vi "pointReactorSimulator.vi"() -> ()   [LabVIEW 2020]
doc: "本程序通过点堆动力学模型模拟核电站的反应堆运行状态。"
uses:
  <vilib>/Instr/_visa.llb/VISA Find Search Mode.ctl
  <vilib>/Utility/sysdir.llb/System Directory Type.ctl
  <vilib>/Utility/error.llb/DialogType.ctl
  Utility/Typedefs/KE622x -- Instrument Type.ctl
  Configure/Source/Typedefs/KE622x -- Voltage Limit.ctl
  Configure/Source/Typedefs/KE622x -- Current Range.ctl
  Configure/Source/Typedefs/KE622x -- Current Ranges.ctl
  <vilib>/DAQmx/write.llb/DAQmx Write (Counter 1D Frequency 1Chan NSamp).vi
  <vilib>/DAQmx/write.llb/DAQmx Write (Analog DBL 1Chan 1Samp).vi
  <vilib>/Analysis/polynomials.llb/Scalar Polynomial Evaluation (DBL).vi
  <vilib>/Instr/_visa.llb/VISA Configure Serial Port (Instr).vi
  <vilib>/DAQmx/create/channels.llb/DAQmx Create Channel (CO-Pulse Generation-Frequency).vi
  <vilib>/DAQmx/configure/timing.llb/DAQmx Timing (Implicit).vi
  <vilib>/DAQmx/create/channels.llb/DAQmx Create Channel (AO-Voltage-Basic).vi
  <vilib>/DAQmx/miscellaneous.llb/DAQmx Fill In Error Info.vi
  TcpModbus_SlaveServer/MB Slave Init (poly).vi
  TcpModbus_SlaveServer/MB Globals.vi
  TcpModbus_SlaveServer/MB Slave Read Holding Registers (poly).vi
  TcpModbus_SlaveServer/MB Slave Write Input Registers (poly).vi
  PointReactorDll.dll
  <vilib>/Analysis/NI_AALPro.lvlib
  Keithley 622x.lvlib
  <resource>/objmgr/daqmx.rc
panel:
  out "KE6220_2":bool
  in  "物理参数设置":bool
  in  "endian Switch":bool
  out "反应性仪输出电压":dbl[](array[numeric])
  out "输出电压":dbl[](array[numeric])
  in  "输出电流 (A)":dbl
  in  "电压输出选择":bool
  out "中子注量率 (n/cm2·s)":dbl
  out "硼总价值 (pcm)":dbl
  out "棒总价值 (pcm)":dbl
  out "硼浓度 indicator":dbl
  in  "硼浓度 (ppm)":dbl(slide)=1.0 scale=0.0..2000.0
  out "运行时间 (s)":dbl
  in  "TCP端口号":u16=502 min=1 max=9999
  out "堆芯反应性(硼+棒) (pcm)":dbl
  out "keff":dbl
  in  "S棒组":dbl(slide)=100.0 min=0.0 max=225.0 scale=0.0..225.0
  in  "A棒组":dbl(slide)=100.0 min=0.0 max=225.0 scale=0.0..225.0
  in  "B棒组":dbl(slide)=100.0 min=0.0 max=225.0 scale=0.0..225.0
  in  "C棒组":dbl(slide)=100.0 min=0.0 max=225.0 scale=0.0..225.0
  in  "堆芯后备反应性 (pcm)":dbl
  out "S棒价值":dbl
  out "A棒价值":dbl
  out "B棒价值":dbl
  out "C棒价值":dbl
  out "D棒价值":dbl
  out "中子注量曲线":dbl(graph) caption="Waveform Chart - Dark"
  in  "D棒组":dbl(slide)=100.0 min=0.0 max=225.0 scale=0.0..225.0
  out "CARD":bool
  out "KE6220_1":bool
  out "COM2":bool
  out "COM1":bool
  in  "VO 4":u16(ring)=3 items=["D棒位 (step)", "C棒位 (step)", "B棒位 (step)", "A棒位 (step)", "S棒位 (step)", "硼浓度 (ppm)", "中间量程电流 (A)", "源量程计数 (CPS)"]
  in  "VO 3":u16(ring)=2 items=["D棒位 (step)", "C棒位 (step)", "B棒位 (step)", "A棒位 (step)", "S棒位 (step)", "硼浓度 (ppm)", "中间量程电流 (A)", "源量程计数 (CPS)"]
  in  "VO 2":u16(ring)=1 items=["D棒位 (step)", "C棒位 (step)", "B棒位 (step)", "A棒位 (step)", "S棒位 (step)", "硼浓度 (ppm)", "中间量程电流 (A)", "源量程计数 (CPS)"]
  in  "VO 1":u16(ring) items=["D棒位 (step)", "C棒位 (step)", "B棒位 (step)", "A棒位 (step)", "S棒位 (step)", "硼浓度 (ppm)", "中间量程电流 (A)", "源量程计数 (CPS)"]
  in  "电信号输出设置":bool
  in  "TCP服务器开":bool
  out "Holding Registers":sgl[](array[numeric]) caption="Holding Registers (Read&Write)"
  out "Coils":bool[](array[boolean]) caption="Coils (Master can write coils)"
  in  "电流输出选择":u16(ring) items=["中间量程电流", "功率量程电流"]
  out "棒位与硼浓度":dbl[](array[numeric])
  in  "反应性控制方式":bool
  in  "归零":bool
  in  "棒速(step/min)":dbl=72.0 min=1.0 max=10000.0 step=1.0 format="%#.3g"
  in  "开始降棒":bool
  in  "降棒选择":u16(ring) items=["D棒组", "C棒组", "B棒组", "A棒组", "S棒组"]
  in  "细分时间 (ms)":u32=100 min=10 max=1000 step=1
  in  "开始":bool
  in  "时间比例尺":dbl(knob)=1.0 min=0.1 max=1000.0 step=0.1 scale=0.1..1000.0
  out "功率量程 (A)":dbl(slide) scale=2.875e-12..0.00023 scale format="%#_6e"
  out "中间量程 (A)":dbl(slide) scale=1e-11..0.0008 scale format="%#_6e"
  out "源量程 (CPS)":dbl(slide) scale=1.0..1000000.0 scale format="%#_6f"
  out "%FP":dbl(slide) scale=2e-09..200.0 scale format="%#_6e"
  out "中子注量率":dbl(slide) scale=0.1..10000000000.0 scale format="%#_6e"
  in  "时间步长 (s)":dbl=0.1
  in  "初始注量率 (n/cm2·s)":dbl=1.0
  in  "堆芯反应性 (pcm)":dbl
  in  "停止":bool
  in  "初始反应性 (pcm)":dbl
  # "反应性仪测试用点堆模拟器"
  # "探测器"
  # "手输"
  # "棒硼"
  # "1.25E+5 n/cm2·s\n——"
  # "——\n1.25E+2 n/cm2·s"
  # "——  1.25E-1 n/cm2·s"
  # "硬件测试"
  # "小端"
  # "0-10V"
  # "1-5V"
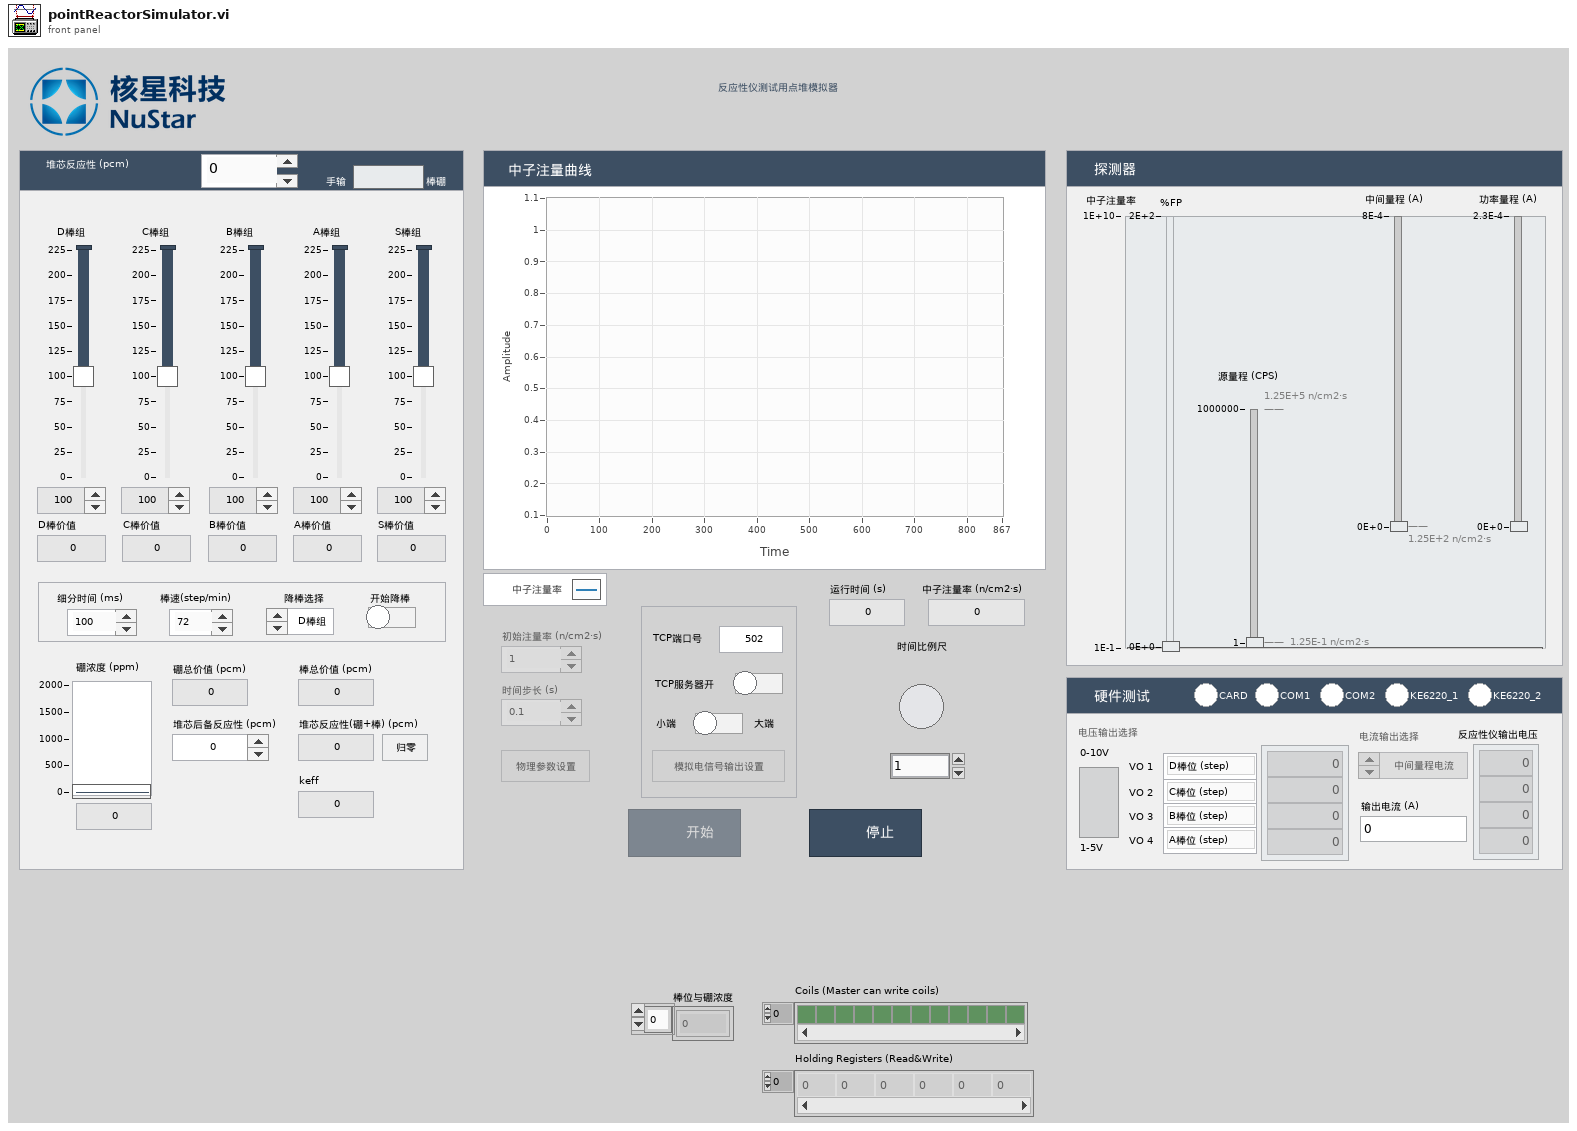
[diagram p1: front panel]
types:
  T1 = enum8{"Enabled", "Disabled", "Disabled and Grayed Out"}
  T2 = typedef "System Directory Type.ctl" = i32
  T3 = typedef "VISA Find Search Mode.ctl" = u32
  T4 = enum16{"open", "open or create", "create or replace", "create", "open (read only)"}
  T5 = typedef "DialogType.ctl" = u16
  T6 = typedef "Keithley 622x.lvlib/KE622x -- Voltage Limit.ctl" = dbl
  T7 = typedef "Keithley 622x.lvlib/KE622x -- Instrument Type.ctl" = enum16{"KE6220", "KE6221"}
  T8 = typedef "Keithley 622x.lvlib/KE622x -- Current Range.ctl" = cluster{"Auto Range?":bool, "Man / Selected\nRange":T9}
  T9 = typedef "Keithley 622x.lvlib/KE622x -- Current Ranges.ctl" = enum16{"2nA", "20nA", "200nA", "2uA", "20uA", "200uA", "2mA", "20mA", "100mA"}
  T10 = enum32{"invalid app kind", "Development System", "Run Time System", "Student Edition", "Embedded LabVIEW", "Evaluation", "Custom"}
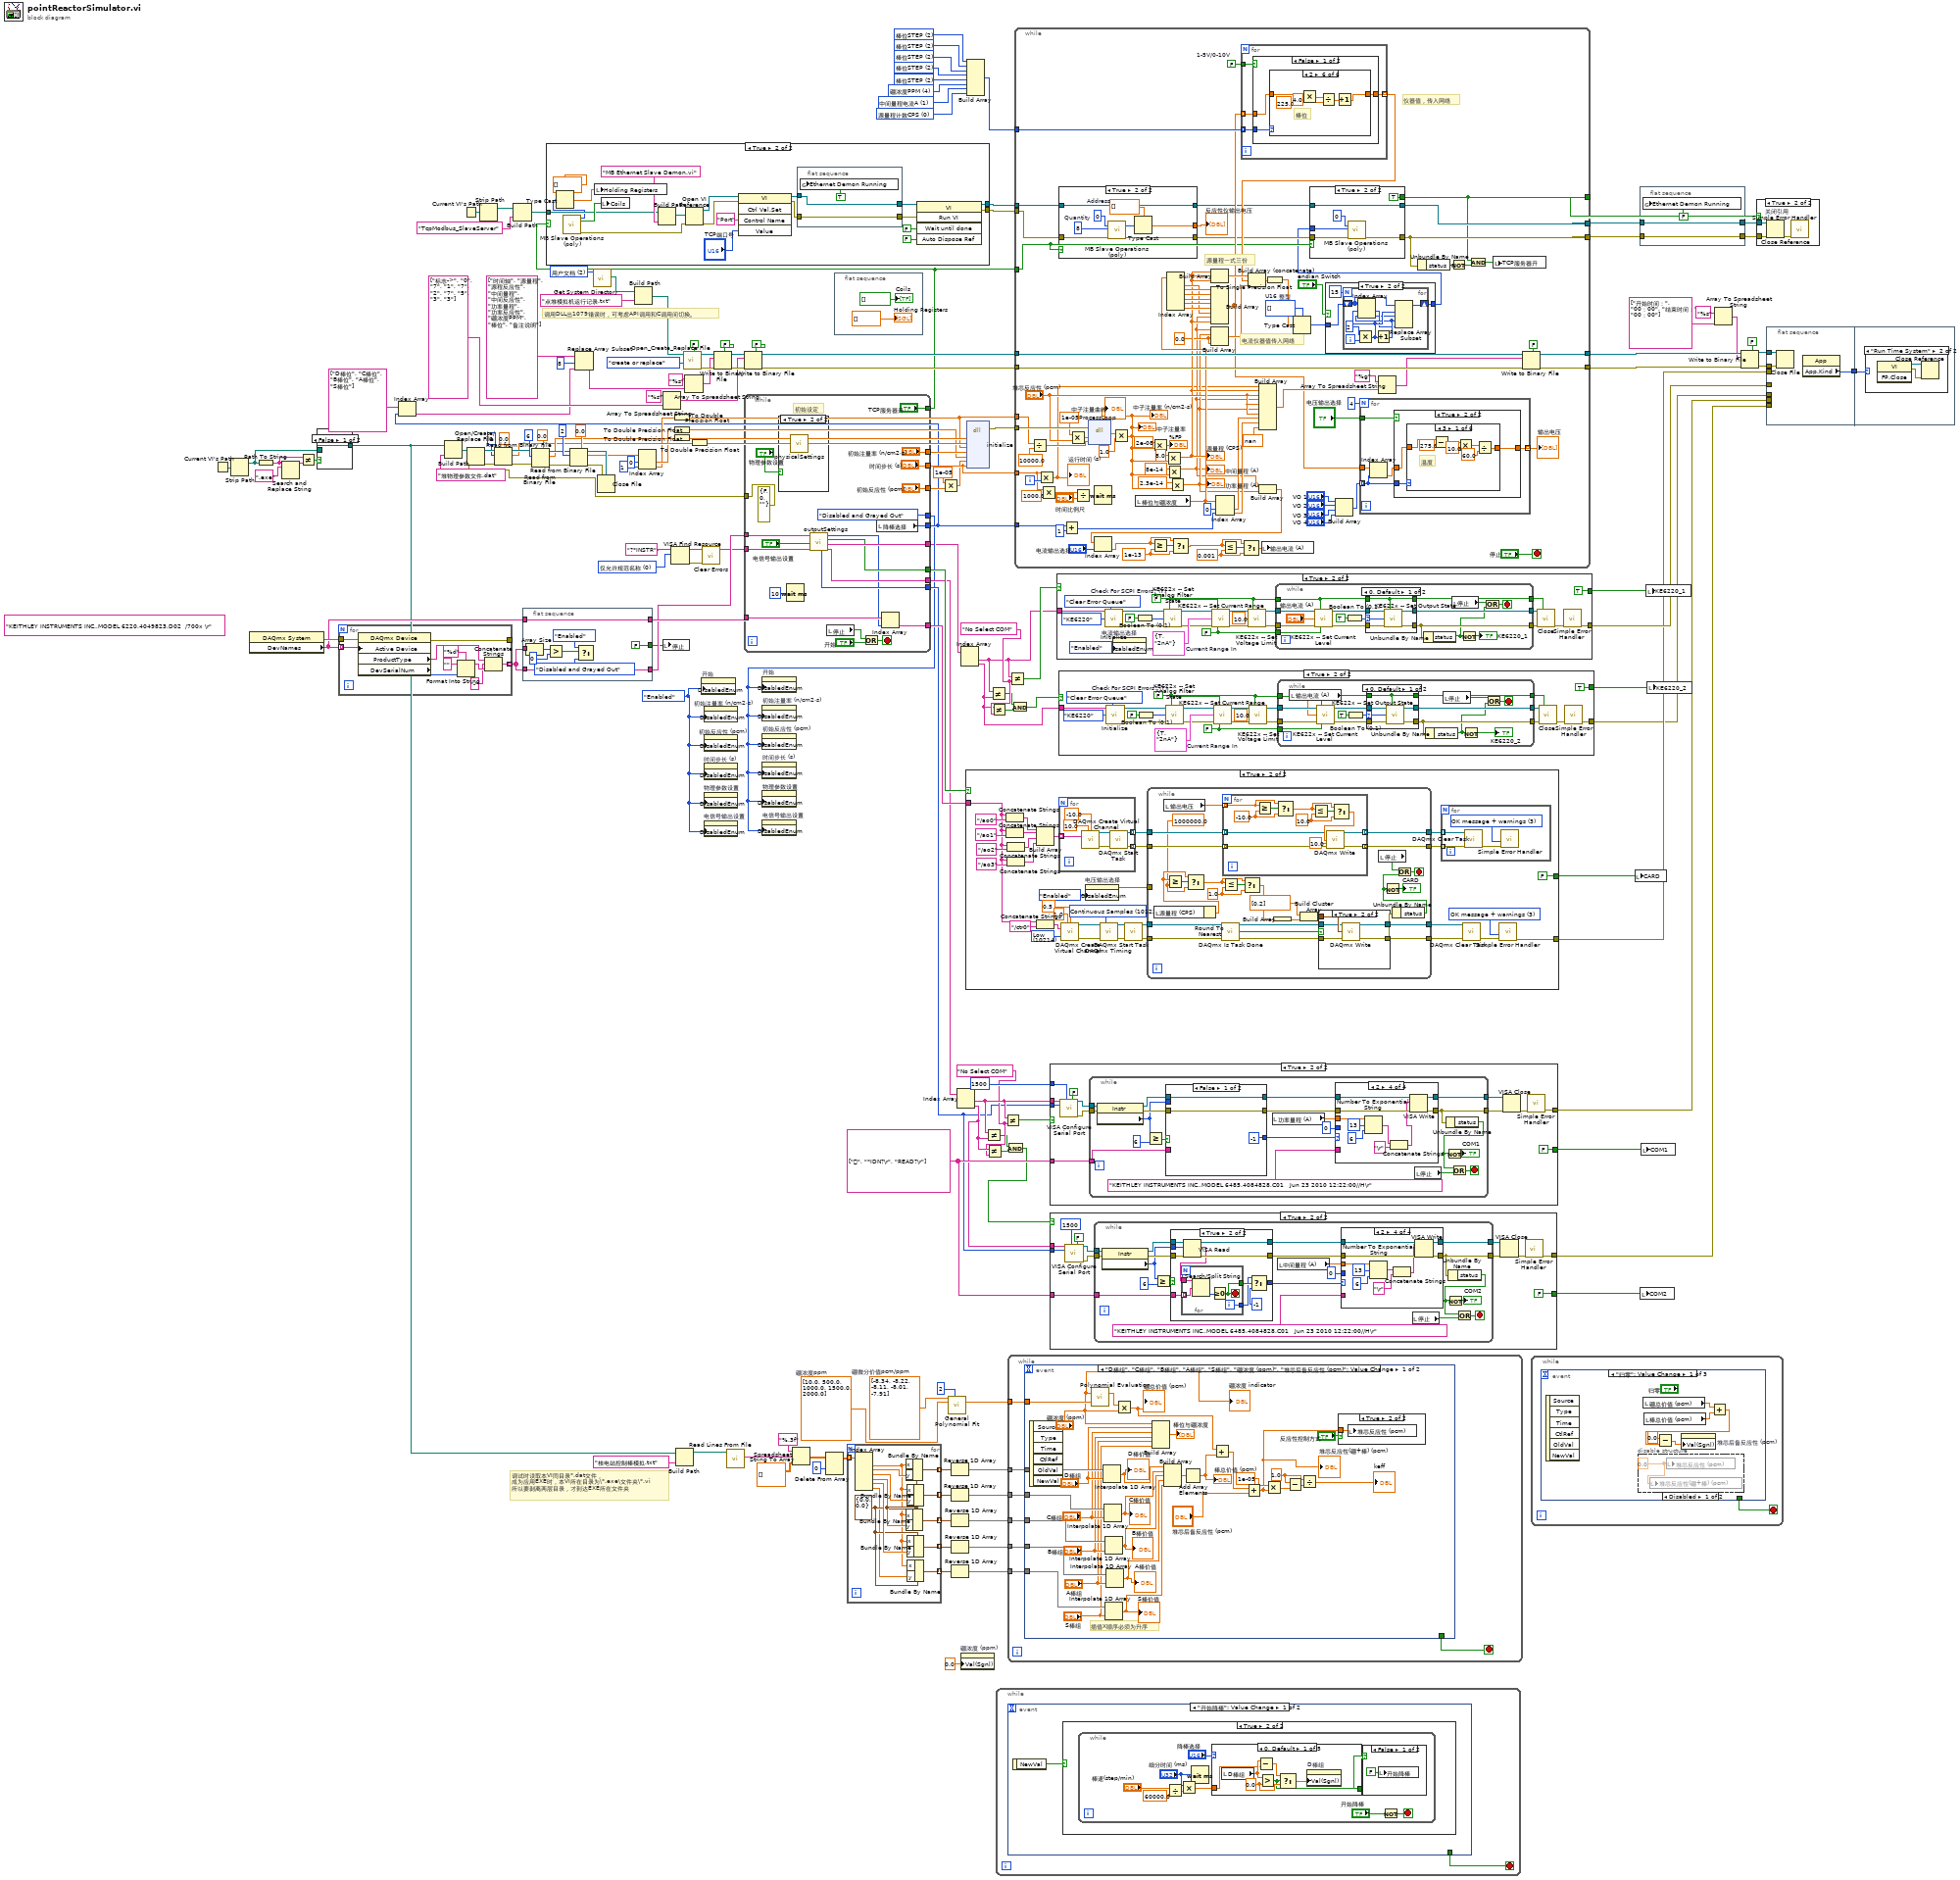
[diagram p0: block diagram]
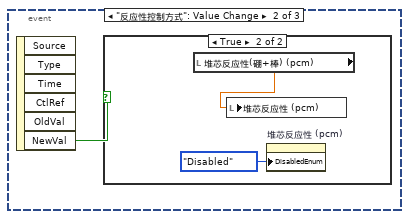
[diagram p3: hidden frame]
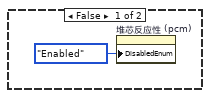
[diagram p4: hidden frame]
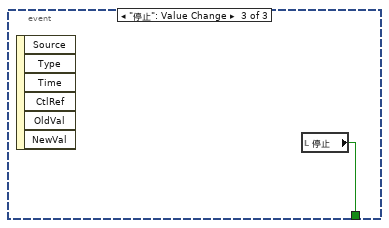
[diagram p5: hidden frame]
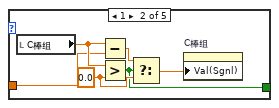
[diagram p8: hidden frame]
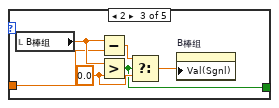
[diagram p9: hidden frame]
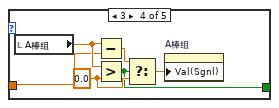
[diagram p10: hidden frame]
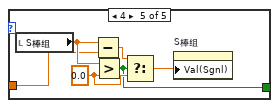
[diagram p11: hidden frame]
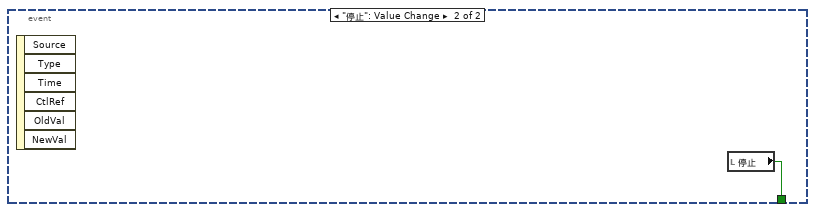
[diagram p12: hidden frame]
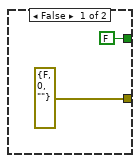
[diagram p13: hidden frame]
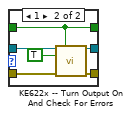
[diagram p14: hidden frame]
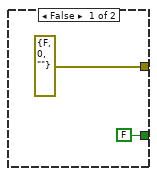
[diagram p15: hidden frame]
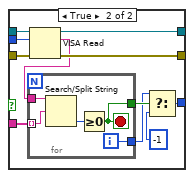
[diagram p16: hidden frame]
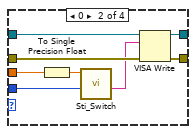
[diagram p18: hidden frame]
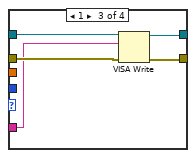
[diagram p19: hidden frame]
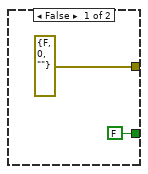
[diagram p20: hidden frame]
diagram:
  w3 = T1."Enabled" ("禁用")
  w11 = "No Select COM" ("新元素/子数组")
  (unwired) "KEITHLEY INSTRUMENTS INC.,MODEL 6220,4049823,D02  /700x \r" ("y")
  w17 = T2 2 items=["用户目录"=0, "用户桌面"=1, "用户文档"=2, "用户应用程序数据"=3, "用户设置"=4, "用户临时目录"=5, "公共文档"=6, "公共应用程序数据"=7, "公共设置"=8, "公共缓存"=13, "系统核心库"=9, "系统安装库"=10, "应用程序文件"=11, "启动盘根目录"=12] ("system directory type")
  w37 = "No Select COM" ("新元素/子数组")
  w42 = string[] ["", "*IDN?\r", "READ?\r"] ("添加的数组")
  w52 = u16 0 items=["源量程计数CPS", "中间量程电流A", "棒位STEP", "温度(摄氏度)", "硼浓度PPM", "P2电压信号"] ("P2-8")
  w51 = u16 1 items=["源量程计数CPS", "中间量程电流A", "棒位STEP", "温度(摄氏度)", "硼浓度PPM", "P2电压信号"] ("P2-7")
  w50 = u16 4 items=["源量程计数CPS", "中间量程电流A", "棒位STEP", "温度(摄氏度)", "硼浓度PPM", "P2电压信号"] ("P2-6")
  w49 = u16 2 items=["源量程计数CPS", "中间量程电流A", "棒位STEP", "温度(摄氏度)", "硼浓度PPM", "P2电压信号"] ("P2-5")
  w48 = u16 2 items=["源量程计数CPS", "中间量程电流A", "棒位STEP", "温度(摄氏度)", "硼浓度PPM", "P2电压信号"] ("P2-4")
  w47 = u16 2 items=["源量程计数CPS", "中间量程电流A", "棒位STEP", "温度(摄氏度)", "硼浓度PPM", "P2电压信号"] ("P2-3")
  w46 = u16 2 items=["源量程计数CPS", "中间量程电流A", "棒位STEP", "温度(摄氏度)", "硼浓度PPM", "P2电压信号"] ("P2-2")
  w45 = u16 2 items=["源量程计数CPS", "中间量程电流A", "棒位STEP", "温度(摄氏度)", "硼浓度PPM", "P2电压信号"] ("P2-1")
  w65 = T3 0 items=["仅允许规范名称"=0, "只允许别名"=2, "包含匹配别名"=3, "包含所有别名"=4] ("Search Mode")
  w91 = dbl[] [-8.34, -8.22, -8.11, -8.01, -7.91]  # 硼微分价值pcm/ppm
  w90 = dbl[] [10.0, 500.0, 1000.0, 1500.0, 2000.0]  # 硼浓度ppm
  # "调试时读取本VI同目录*.dat文件，\n成为应用EXE时，本VI所在目录为\\*.exe\\文件夹\\*.vi\n所以要剥离两层目录，才到达EXE所在文件夹"
  # "调用DLL出1079错误时，可考虑API调用和C调用间切换。"
  n1 = Current VI's Path() -> (path=w125:path)
  n2 = Strip Path(path=w125) -> (stripped path=w120:path)  [unwired: 1 out]
  n3 = property class="DAQmx System"() -> (error out=w71:errorcluster, "DevNames"=w69:tag[])  [unwired: 2 in, 1 out]
  n4 = Path To String(path=w120) -> (string=w122:string)
  n5 = Search and Replace String(input string=w122, search string=".exe" ("搜索字符串")) -> (result string=w123:string)  [unwired: 6 in, 3 out]
  n6 = Not Equal?(x=w122, y=w123) -> (x != y?=w121:bool)
  n7 = case shown="False" w121 {
    tunnel: w120 -> [w163 w165]
    tunnel: [w163 w164] -> w19
    frame False {
    }
    frame True {
      n8 = Strip Path(path=w165) -> (stripped path=w164:path)  [unwired: 1 out]
    }
  }
  n9 = for {
    tunnel: w69 -> [w175] mode=indexing
    tunnel: w71 -> [w174]
    tunnel: [w173] -> _
    tunnel: [w166] -> w70 mode=indexing
    n10 = property class="DAQmx Device"(error in=w174, "Active Device"=w175) -> (error out=w173:errorcluster, "ProductType"=w169:string, "DevSerialNum"=w170:u32)  [unwired: 1 in, 1 out]
    n11 = Format Into String(format string="%d" ("格式字符串"), initial string="" ("初始字符串"), w170) -> (resulting string=w168:string)  [unwired: 1 in, 1 out]
    n12 = Concatenate Strings(w169, "-" ("字符串"), w168) -> (w166:string)
  }
  n13 = Build Path(base path=w19, name or relative path="堆物理参数文件.dat") -> (appended path=w126:path)
  n14 = Current VI's Path() -> (path=w57:path)
  n15 = Strip Path(path=w57) -> (stripped path=w56:path)  [unwired: 1 out]
  n16 = Build Path ("创建路径")(base path=w56, name or relative path="TcpModbus_SlaveServer" ("搜索字符串")) -> (appended path=w55:path)
  n17 = flat-sequence {
    tunnel: w70 -> [w184]
    tunnel: [w179] -> w43
    tunnel: w70 -> [w179]
    tunnel: w69 -> [w178]
    tunnel: [w178] -> w68
    tunnel: [FALSE ("停止")] -> w28
    frame #0 {
      n18 = Array Size(array=w184) -> (size(s)=w183:i32)
      n19 = Greater?(x=w183, y=0) -> (0:w180:bool)
      n20 = Select(t=T1."Enabled" ("禁用"), s=w180, f=T1."Disabled and Grayed Out" ("禁用")) -> ()  [unwired: 1 out]
    }
  }
  n21 = call <vilib>:"Get System Directory.vi"("system directory type"=w17) -> ("system directory"=w18:path)  [unwired: 10 in]
  n22 = Build Path(base path=w18, name or relative path="点堆模拟机运行记录.txt") -> (appended path=w135:path)
  n23 = local write "停止"(w28) -> ()
  n24 = Array To Spreadsheet String(array=string[] ["标志->", "0", "7", "1", "7", "2", "7", "5", "3", "3"] ("添加的数组"), 3:"%s" ("format string")) -> (spreadsheet string=w148:string)  [unwired: 1 in]
  n25 = VISA Find Resource(10:w65, 11:"?*INSTR" ("表达式(\"?*\")")) -> (0:w58:errorcluster, 3:w14:string[])  [unwired: 1 in, 1 out]
  n26 = Build Path(base path=w19, name or relative path="核电站控制棒模拟.txt") -> (appended path=w108:path)
  n27 = call <vilib>:"Open_Create_Replace File.vi"("advisory dialog? (display:T)"=FALSE, "function (open:0)"=T4."create or replace", "file path"=w135) -> ("error out"=w155:errorcluster, "refnum"=w156:refnum<file>)  [unwired: 5 in, 2 out]
  n28 = property on="开始" class="Bool"("DisabledEnum"=w3) -> ()  [unwired: 2 in, 2 out]
  n29 = call <vilib>:"Clear Errors.vi"("error in (no error)"=w58) -> ()  [unwired: 5 in, 2 out]
  n30 = property on="初始注量率 (n/cm2·s)" class="DigNum (strict)"("DisabledEnum"=w3) -> ()  [unwired: 2 in, 2 out]
  n31 = property on="初始反应性 (pcm)" class="DigNum (strict)"("DisabledEnum"=w3) -> ()  [unwired: 2 in, 2 out]
  n32 = property on="时间步长 (s)" class="DigNum (strict)"("DisabledEnum"=w3) -> ()  [unwired: 2 in, 2 out]
  n33 = property on="物理参数设置" class="Bool"("DisabledEnum"=w3) -> ()  [unwired: 2 in, 2 out]
  n34 = property on="电信号输出设置" class="Bool"("DisabledEnum"=w3) -> ()  [unwired: 2 in, 2 out]
  n35 = call <vilib>:"Read Lines From File.vi"("file path (dialog if empty)"=w108) -> ("line string"=w105:string)  [unwired: 5 in, 3 out]
  n36 = while {
    tunnel: ["初始注量率 (n/cm2·s)"] -> w161
    tunnel: ["时间步长 (s)"] -> w160
    tunnel: ["初始反应性 (pcm)"] -> w132
    tunnel: [w200] -> w63
    tunnel: [w196] -> w8
    tunnel: [w195] -> w72
    tunnel: w68 -> [w203]
    tunnel: [w202] -> w67
    tunnel: ["TCP服务器开"] -> w60
    tunnel: w14 -> [w198]
    tunnel: [w193] -> w53
    tunnel: [w197] -> w33
    tunnel: w43 -> [w199]
    tunnel: [T1."Disabled and Grayed Out" ("禁用")] -> w15
    tunnel: [errorcluster {"status"=FALSE, "code"=0, "source"=""} ("error in")] -> w16
    stop <- w189 stop-if-true
    # "初始设定"
    n37 = case shown="True" "物理参数设置" {
      frame False {
      }
      frame True {
        n38 = call "physicalSettings.vi"() -> ()  [unwired: 1 in]
      }
    }
    n39 = Wait (ms)(milliseconds to wait=u32 10) -> ()  [unwired: 1 out]
    n40 = call "outputSettings.vi"("所有串口"=w198, "执行:调用时显示前面板"="电信号输出设置", "电压脉冲卡选择"=w199) -> ("串口电流服务选定口"=w193:string[], "电流源串口选定"=w196:string[], "电压脉冲开关 2"=w195:bool, "电压脉冲卡选"=w192:u16, "波特率set"=w197:u32)  [unwired: 4 in]
    n41 = local read "停止"() -> (w191:bool)
    n42 = Or(x=w191, y="开始") -> (x .or. y?=w189:bool)
    n43 = local read "降棒选择"() -> (w200:u16)
    n44 = Index Array(array=w203, index=w192) -> (element=w202:tag)
  }
  n45 = Index Array(array=string[] ["D棒位", "C棒位", "B棒位", "A棒位", "S棒位"] ("添加的数组"), index=w63) -> (element=w74:string)
  n46 = Open/Create/Replace File(file path (use dialog)=w126, error in=w16) -> (refnum out=w131:refnum<file>, error out=w130:errorcluster)  [unwired: 4 in, 1 out]
  n47 = Read from Binary File(5:sgl 0.0 ("byte stream type"), 8:w130, 10:6 ("count"), 11:w131) -> (0:w116:errorcluster, 2:w82:sgl[], 3:w117:refnum<file>)  [unwired: 2 in, 1 out]
  n48 = Read from Binary File(5:sgl 0.0 ("byte stream type"), 8:w116, 10:6 ("count"), 11:w117) -> (0:w112:errorcluster, 2:w84:sgl[], 3:w113:refnum<file>)  [unwired: 2 in, 1 out]
  n49 = case shown="True" w60 {
    tunnel: [refnum<vi> refnum w216] -> w62
    tunnel: [errorcluster {"status"=FALSE, "code"=0, "source"=""} ("error out") w215] -> w61
    tunnel: w55 -> [_ w214]
    frame False {
    }
    frame True {
      n50 = call-poly "MB Slave Operations (poly).vi"() -> ("Holding Registers"=w213:u16[], "Coils"=w224:bool[], "error out"=w222:errorcluster)  [unwired: 1 in, 16 out]
      n51 = Type Cast(type=sgl[] [] ("添加的数组"), x=w213) -> (*(type *) &x=w212:sgl[])
      n52 = local write "Holding Registers"(w212) -> ()
      n53 = local write "Coils"(w224) -> ()
      n54 = Build Path ("创建路径")(base path=w214, name or relative path="MB Ethernet Slave Demon.vi") -> (appended path=w210:path)
      n55 = Open VI Reference(vi path=w210, error in (no error)=w222) -> (vi reference=w219:refnum<vi>, error out=w220:errorcluster)  [unwired: 4 out]
      n56 = invoke class="VI" method="Ctrl Val.Set"(reference=w219, error in=w220, "Control Name"="Port", "Value"="TCP端口号") -> (reference out=w227:refnum<vi>, error out=w226:errorcluster)  [unwired: 1 in, 3 out]
      n57 = flat-sequence {
        tunnel: [w231] -> w223
        tunnel: w226 -> [w231]
        tunnel: [w229] -> w225
        tunnel: w227 -> [w229]
        frame #0 {
          n58 = global write "MB Globals.vi" "Ethernet Demon Running"(TRUE ("Slave Demon Running")) -> ()
        }
      }
      n59 = invoke class="VI" method="Run VI"(reference=w225, error in=w223, "Wait until done"=FALSE, "Auto Dispose Ref"=FALSE) -> (reference out=w216:refnum<vi>, error out=w215:errorcluster)  [unwired: 1 in, 3 out]
    }
  }
  n60 = Read from Binary File(5:sgl 0.0 ("byte stream type"), 8:w112, 10:2 ("count"), 11:w113) -> (0:w110:errorcluster, 2:w87:sgl[], 3:w111:refnum<file>)  [unwired: 2 in, 1 out]
  n61 = Replace Array Subset(array=string[] ["时间轴", "源量程", "源程反应性", "中间量程", "中间反应性", "功率量程", "功率反应性", "硼浓度PPM", "棒位", "备注说明"] ("添加的数组"), new element=w74, index=8 ("索引")) -> (w73:string[])
  n62 = Close File(refnum=w111, error in=w110) -> ()  [unwired: 2 out]
  n63 = Index Array(array=w87, index #1=0 ("索引"), index #2=1 ("索引")) -> (element #1=w80:sgl, element #2=w78:sgl)
  n64 = To Double Precision Float(number=w78) -> (double precision float=w77:dbl)
  n65 = To Double Precision Float(number=w80) -> (double precision float=w79:dbl)
  n66 = To Double Precision Float(number=w84) -> (double precision float=w83:dbl[])
  n67 = Array To Spreadsheet String(array=w73, 3:"%s" ("format string")) -> (spreadsheet string=w153:string)  [unwired: 1 in]
  n68 = To Double Precision Float(number=w82) -> (double precision float=w81:dbl[])
  n69 = Write to Binary File(file (use dialog)=w156, data=w153, error in=w155, 5:FALSE ("预置数组或字符串大小？(T)")) -> (refnum out=w151:refnum<file>, error out=w150:errorcluster)  [unwired: 2 in, 1 out]
  n70 = Write to Binary File(file (use dialog)=w151, data=w148, error in=w150, 5:FALSE ("预置数组或字符串大小？(T)")) -> (refnum out=w146:refnum<file>, error out=w145:errorcluster)  [unwired: 2 in, 1 out]
  n71 = property on="开始" class="Bool"("DisabledEnum"=w15) -> ()  [unwired: 2 in, 2 out]
  n72 = property on="初始注量率 (n/cm2·s)" class="DigNum (strict)"("DisabledEnum"=w15) -> ()  [unwired: 2 in, 2 out]
  n73 = property on="初始反应性 (pcm)" class="DigNum (strict)"("DisabledEnum"=w15) -> ()  [unwired: 2 in, 2 out]
  n74 = property on="时间步长 (s)" class="DigNum (strict)"("DisabledEnum"=w15) -> ()  [unwired: 2 in, 2 out]
  n75 = property on="物理参数设置" class="Bool"("DisabledEnum"=w15) -> ()  [unwired: 2 in, 2 out]
  n76 = property on="电信号输出设置" class="Bool"("DisabledEnum"=w15) -> ()  [unwired: 2 in, 2 out]
  n77 = Spreadsheet String To Array ("电子表格字符串至数组转换")(format string="%.3f" ("format (%.3f)"), spreadsheet string=w105, array type (2D Dbl)=dbl[][] [] ("type (empty)")) -> (array=w104:dbl[][])  [unwired: 1 in]
  n78 = Delete From Array(array=w104, index (row)=0 ("索引 (行)")) -> (array with subset deleted=w102:dbl[][])  [unwired: 2 in, 1 out]
  n79 = flat-sequence {
    frame #0 {
      "Coils" <- bool[] [] ("Coils")
      "Holding Registers" <- sgl[] [] ("Holding Registers")
    }
  }
  n80 = for {
    tunnel: w102 -> [w246] mode=indexing
    tunnel: [w244] -> w101 mode=indexing
    tunnel: [w240] -> w99 mode=indexing
    tunnel: [w239] -> w98 mode=indexing
    tunnel: [w238] -> w97 mode=indexing
    tunnel: [w236] -> w93 mode=indexing
    w237 = cluster{"x":dbl, "y":dbl} {"x"=0.0, "y"=0.0} ("输入簇")
    n81 = Index Array(array=w246) -> (element #1=w234:dbl, element #2=w245:dbl, element #3=w243:dbl, element #4=w242:dbl, element #5=w241:dbl, element #6=w235:dbl)  [unwired: 6 in]
    n82 = Bundle By Name(cluster=w237, "x"=w234, "y"=w245) -> (w244:cluster{"x":dbl, "y":dbl})
    n83 = Bundle By Name(cluster=w237, "x"=w234, "y"=w242) -> (w239:cluster{"x":dbl, "y":dbl})
    n84 = Bundle By Name(cluster=w237, "x"=w234, "y"=w243) -> (w240:cluster{"x":dbl, "y":dbl})
    n85 = Bundle By Name(cluster=w237, "x"=w234, "y"=w241) -> (w238:cluster{"x":dbl, "y":dbl})
    n86 = Bundle By Name(cluster=w237, "x"=w234, "y"=w235) -> (w236:cluster{"x":dbl, "y":dbl})
  }
  n87 = Multiply(x=1e-05, y=w132) -> (x*y=w133:dbl)
  n88 = call <vilib>:"General Polynomial Fit.vi"("Y"=w91, "polynomial order"=2, "X"=w90) -> ("Polynomial Coefficients"=w88:dbl[])  [unwired: 9 in, 3 out]
  n89 = Reverse 1D Array(array=w101) -> (reversed array=w100:cluster{"x":dbl, "y":dbl}[])
  n90 = Reverse 1D Array(array=w99) -> (reversed array=w96:cluster{"x":dbl, "y":dbl}[])
  n91 = Reverse 1D Array(array=w98) -> (reversed array=w95:cluster{"x":dbl, "y":dbl}[])
  n92 = Reverse 1D Array(array=w97) -> (reversed array=w94:cluster{"x":dbl, "y":dbl}[])
  n93 = Reverse 1D Array(array=w93) -> (reversed array=w92:cluster{"x":dbl, "y":dbl}[])
  n94 = Index Array(array=w53) -> (element #1=w40:string, element #2=w38:string)  [unwired: 2 in]
  n95 = property on="硼浓度 (ppm)" class="Slide (strict)"("Val(Sgnl)"=0.0 ("Value (Signaling)")) -> ()  [unwired: 2 in, 2 out]
  n96 = Index Array(array=w8) -> (element #1=w6:string, element #2=w4:string)  [unwired: 2 in]
  n97 = case shown="True" w72 {
    tunnel: w67 -> [_ w250]
    tunnel: [errorcluster {"status"=FALSE, "code"=0, "source"=""} ("error out") w252] -> w31
    tunnel: [FALSE ("停止") FALSE ("停止")] -> w24
    frame False {
      n98 = property on="电压输出选择" class="Bool (strict)"("DisabledEnum"=T1."Disabled and Grayed Out" ("禁用")) -> ()  [unwired: 2 in, 2 out]
    }
    frame True {
      w269 = 10214 items=["High"=10192, "Low"=10214] ("Idle State")
      w268 = 10123 items=["Finite Samples"=10178, "Continuous Samples"=10123] ("sample mode")
      w273 = T5 3 items=["no dialog", "OK message", "continue or stop message", "OK message + warnings", "continue/stop + warnings"] ("type of dialog (OK msg:1)")
      n99 = Concatenate Strings(w250, "/ao0") -> (w257:string)
      n100 = Concatenate Strings(w250, "/ao1") -> (w256:string)
      n101 = Concatenate Strings(w250, "/ao2") -> (w255:string)
      n102 = Concatenate Strings(w250, "/ao3") -> (w254:string)
      n103 = Concatenate Strings(w250, "/ctr0") -> (w261:string)
      n104 = Build Array(w257, w256, w255, w254) -> (w253:string[])
      n105 = for {
        tunnel: [w290] -> w279 mode=indexing
        tunnel: [w289] -> w278 mode=indexing
        tunnel: w253 -> [w288] mode=indexing
        n106 = call-poly <vilib>:"DAQmx Create Virtual Channel.vi"("maximum value"=10.0 ("Maximum Value"), "minimum value"=-10.0 ("Minimum Value"), "physical channels"=w288) -> ("task out"=w292:refnum<k21>, "error out"=w291:errorcluster)  [unwired: 11 in]
        n107 = call <vilib>:"DAQmx Start Task.vi"("task/channels in"=w292, "error in"=w291) -> ("task out"=w290:refnum<k21>, "error out"=w289:errorcluster)  [unwired: 12 in]
      }
      n108 = call-poly <vilib>:"DAQmx Create Virtual Channel.vi"("frequency"=1.0 ("duty cycle"), "duty cycle"=0.5, "counter"=w261, "idle state"=w269) -> ("task out"=w265:refnum<k21>, "error out"=w264:errorcluster)  [unwired: 10 in]
      n109 = property on="电压输出选择" class="Bool (strict)"("DisabledEnum"=T1."Enabled" ("禁用")) -> (error out=w276:errorcluster)  [unwired: 2 in, 1 out]
      n110 = call-poly <vilib>:"DAQmx Timing.vi"("task/channels in"=w265, "sample mode"=w268, "error in"=w264) -> ("task out"=w267:refnum<k21>, "error out"=w266:errorcluster)  [unwired: 11 in]
      n111 = call <vilib>:"DAQmx Start Task.vi"("task/channels in"=w267, "error in"=w266) -> ("task out"=w263:refnum<k21>, "error out"=w262:errorcluster)  [unwired: 12 in]
      n112 = while {
        tunnel: [w321] -> w282
        tunnel: [w320] -> w281
        tunnel: w279 -> [w319]
        tunnel: w278 -> [w318]
        tunnel: [w309] -> w275
        tunnel: [w305] -> w274
        tunnel: w263 -> [w300]
        tunnel: w276 -> [_]
        tunnel: w262 -> [w299]
        stop <- w302 stop-if-true
        w311 = 1000000.0 ("y")
        w314 = 1.0 ("y")
        n113 = local read "源量程 (CPS)"() -> (w317:dbl)
        n114 = local read "输出电压"() -> (w295:dbl[])
        n115 = Round To Nearest(number=w317) -> (nearest integer value=w312:dbl)
        n116 = Greater Or Equal?(x=w312, y=w311) -> (x >= y?=w316:bool)
        n117 = Select(t=w312, s=w316, f=w311) -> (s? t:f=w313:dbl)
        n118 = call <vilib>:"DAQmx Is Task Done.vi"("task/channels in"=w300, "error in"=w299) -> ("task out"=w298:refnum<k21>, "task done?"=w296:bool, "error out"=w297:errorcluster)  [unwired: 11 in]
        n119 = Less Or Equal?(x=w313, y=w314) -> (x <= y?=w315:bool)
        n120 = for {
          tunnel: [w339] -> w321 mode=indexing
          tunnel: [w338] -> w320 mode=indexing
          tunnel: w319 -> [w331] mode=indexing
          tunnel: w318 -> [w330] mode=indexing
          tunnel: w295 -> [w329] mode=indexing
          w334 = 10.0 ("y")
          w336 = -10.0 ("y")
          n121 = Greater Or Equal?(x=w329, y=w336) -> (x >= y?=w337:bool)
          n122 = Select(t=w329, s=w337, f=w336) -> (s? t:f=w333:dbl)
          n123 = Less Or Equal?(x=w333, y=w334) -> (x <= y?=w335:bool)
          n124 = Select(t=w333, s=w335, f=w334) -> (s? t:f=w332:dbl)
          n125 = call-poly <vilib>:"DAQmx Write.vi"("task/channels in"=w331, "data"=w332, "timeout"=10.0, "error in"=w330) -> ("task out"=w339:refnum<k21>, "error out"=w338:errorcluster)  [unwired: 9 in, 1 out]
        }
        n126 = Select(t=w313, s=w315, f=w314) -> (s? t:f=w306:dbl)
        n127 = Build Array(w306) -> (w307:dbl[])
        n128 = Build Cluster Array(dbl[] [0.2] ("数组"), w307) -> (w310:cluster{"initial delay":dbl, "y":dbl}[])
        n129 = case shown="True" w296 {
          tunnel: w310 -> [_ w328]
          tunnel: [w323 w327] -> w309
          tunnel: [w322 w326] -> w305
          tunnel: w298 -> [w323 w325]
          tunnel: w297 -> [w322 w324]
          frame False {
          }
          frame True {
            n130 = call-poly <vilib>:"DAQmx Write.vi"("task/channels in"=w325, "data"=w328, "error in"=w324) -> ("task out"=w327:refnum<k21>, "error out"=w326:errorcluster)  [unwired: 10 in, 1 out]
          }
        }
        n131 = local read "停止"() -> (w301:bool)
        n132 = Unbundle By Name(w305) -> ("status"=w303:bool)
        n133 = Not(x=w303) -> (.not. x?=→"CARD":bool)
        n134 = Or(x=w301, y=w303) -> (x .or. y?=w302:bool)
      }
      n135 = for {
        tunnel: w282 -> [w285] mode=indexing
        tunnel: w281 -> [w284] mode=indexing
        w286 = T5 3 items=["no dialog", "OK message", "continue or stop message", "OK message + warnings", "continue/stop + warnings"] ("type of dialog (OK msg:1)")
        n136 = call <vilib>:"DAQmx Clear Task.vi"("task in"=w285, "error in"=w284) -> ("error out"=w287:errorcluster)  [unwired: 13 in]
        n137 = call <vilib>:"Simple Error Handler.vi"("type of dialog (OK msg:1)"=w286, "error in (no error)"=w287) -> ()  [unwired: 3 in, 5 out]
      }
      n138 = call <vilib>:"DAQmx Clear Task.vi"("task in"=w275, "error in"=w274) -> ("error out"=w272:errorcluster)  [unwired: 13 in]
      n139 = call <vilib>:"Simple Error Handler.vi"("type of dialog (OK msg:1)"=w273, "error in (no error)"=w272) -> ("error out"=w252:errorcluster)  [unwired: 3 in, 4 out]
    }
  }
  n140 = Build Array(w45, w46, w47, w48, w49, w50, w51, w52) -> (w44:u16[])
  n141 = dll-call lib="D:/LVprojects/PointReactorSimulator/PointReactorDll.dll" fn="initialize"("lamd"=w83, "bet"=w81, "source"=w77, "n0"=w161, "nlife"=w79, "reactivity"=w133, "delt"=w160) -> (error out=w162:errorcluster)  [unwired: 3 in, 9 out]
  n142 = Not Equal?(x=w40, y=w38) -> (x != y?=w35:bool)
  n143 = Not Equal?(x=w38, y=w37) -> (x != y?=w36:bool)
  n144 = Not Equal?(x=w6, y=w4) -> (x != y?=w9:bool)
  n145 = Not Equal?(x=w4, y=w11) -> (x != y?=w10:bool)
  n146 = while {
    stop <- w341 stop-if-true
    n147 = event shown="[0] \"开始降棒\": Value Change" {
      selector: _ -> [_ _]
      dyn-events: _ -> [_ _]
      timeout: _ -> [_ _]
      tunnel: [_ w383] -> w341
      event "开始降棒": Value Change {
        n148 = event-data() -> ("NewVal"=w342:bool)  [unwired: 1 in]
        n149 = case shown="True" w342 {
          frame False {
          }
          frame True {
            n150 = while {
              stop <- w345 stop-if-true
              n151 = Divide(x="棒速(step/min)", y=60000.0) -> (x/y=w348:dbl)
              n152 = Multiply(x="细分时间 (ms)", y=w348) -> (x*y=w347:dbl)
              n153 = Wait (ms)(milliseconds to wait="细分时间 (ms)") -> ()  [unwired: 1 out]
              n154 = case shown="0, Default" "降棒选择" {
                tunnel: w347 -> [w357 w361 w367 w373 w379]
                tunnel: [w354 w360 w366 w372 w378] -> w343
                frame 0, Default {
                  w355 = 0.0 ("y")
                  n155 = local read "D棒组"() -> (w358:dbl)
                  n156 = Subtract(x=w358, y=w357) -> (x-y=w356:dbl)
                  n157 = Greater?(x=w358, y=w355) -> (0:w354:bool)
                  n158 = Select(t=w356, s=w354, f=w355) -> (s? t:f=w353:dbl)
                  n159 = property on="D棒组" class="Slide (strict)"("Val(Sgnl)"=w353) -> ()  [unwired: 2 in, 2 out]
                }
                frame 1 {
                  w363 = 0.0 ("y")
                  n160 = local read "C棒组"() -> (w362:dbl)
                  n161 = Subtract(x=w362, y=w361) -> (x-y=w364:dbl)
                  n162 = Greater?(x=w362, y=w363) -> (0:w360:bool)
                  n163 = Select(t=w364, s=w360, f=w363) -> (s? t:f=w359:dbl)
                  n164 = property on="C棒组" class="Slide (strict)"("Val(Sgnl)"=w359) -> ()  [unwired: 2 in, 2 out]
                }
                frame 2 {
                  w369 = 0.0 ("y")
                  n165 = local read "B棒组"() -> (w368:dbl)
                  n166 = Subtract(x=w368, y=w367) -> (x-y=w370:dbl)
                  n167 = Greater?(x=w368, y=w369) -> (0:w366:bool)
                  n168 = Select(t=w370, s=w366, f=w369) -> (s? t:f=w365:dbl)
                  n169 = property on="B棒组" class="Slide (strict)"("Val(Sgnl)"=w365) -> ()  [unwired: 2 in, 2 out]
                }
                frame 3 {
                  w375 = 0.0 ("y")
                  n170 = local read "A棒组"() -> (w374:dbl)
                  n171 = Subtract(x=w374, y=w373) -> (x-y=w376:dbl)
                  n172 = Greater?(x=w374, y=w375) -> (0:w372:bool)
                  n173 = Select(t=w376, s=w372, f=w375) -> (s? t:f=w371:dbl)
                  n174 = property on="A棒组" class="Slide (strict)"("Val(Sgnl)"=w371) -> ()  [unwired: 2 in, 2 out]
                }
                frame 4 {
                  w382 = 0.0 ("y")
                  n175 = local read "S棒组"() -> (w380:dbl)
                  n176 = Subtract(x=w380, y=w379) -> (x-y=w381:dbl)
                  n177 = Greater?(x=w380, y=w382) -> (0:w378:bool)
                  n178 = Select(t=w381, s=w378, f=w382) -> (s? t:f=w377:dbl)
                  n179 = property on="S棒组" class="Slide (strict)"("Val(Sgnl)"=w377) -> ()  [unwired: 2 in, 2 out]
                }
              }
              n180 = case shown="False" w343 {
                frame False {
                  n181 = local write "开始降棒"(FALSE ("开始降棒")) -> ()
                }
                frame True {
                }
              }
              n182 = Not(x="开始降棒") -> (.not. x?=w345:bool)
            }
          }
        }
      }
      event "停止": Value Change {
        n183 = event-data() -> ()  [unwired: 1 in, 6 out]
        n184 = local read "停止"() -> (w383:bool)
      }
    }
  }
  n185 = Not Equal?(x=w40, y=w37) -> (x != y?=w39:bool)
  n186 = And(x=w35, y=w36) -> (x .and. y?=w34:bool)
  n187 = while {
    tunnel: w100 -> [w390]
    tunnel: w96 -> [w389]
    tunnel: w95 -> [w388]
    tunnel: w94 -> [w387]
    tunnel: w92 -> [w386]
    tunnel: w88 -> [w385]
    stop <- w384 stop-if-true
    n188 = event shown="[0] \"D棒组\", \"C棒组\", \"B棒组\", \"A棒组\", \"S棒组\", \"硼浓度 (ppm)\", \"堆芯后备反应性 (pcm)\": Value Change" {
      selector: _ -> [_ _]
      dyn-events: _ -> [_ _]
      timeout: _ -> [_ _]
      tunnel: w390 -> [w421 _]
      tunnel: w389 -> [w420 _]
      tunnel: w388 -> [w419 _]
      tunnel: w387 -> [w418 _]
      tunnel: w386 -> [w413 _]
      tunnel: w385 -> [w411 _]
      tunnel: [_ w423] -> w384
      event "D棒组", "C棒组", "B棒组", "A棒组", "S棒组", "硼浓度 (ppm)", "堆芯后备反应性 (pcm)": Value Change {
        w412 = 1.0 ("x")
        # "插值X顺序必须为升序"
        n189 = event-data() -> ()  [unwired: 1 in, 6 out]
        n190 = call-poly <vilib>:"Polynomial Evaluation.vi"("P(x)"=w411, "a"="硼浓度 (ppm)") -> ("P(a)"=w410:dbl)  [unwired: 1 out]
        n191 = Interpolate 1D Array(1:"D棒组", 2:w421) -> (0:w406:dbl)
        "D棒价值" <- w406
        n192 = Interpolate 1D Array(1:"C棒组", 2:w420) -> (0:w405:dbl)
        "C棒价值" <- w405
        n193 = Interpolate 1D Array(1:"B棒组", 2:w419) -> (0:w404:dbl)
        "B棒价值" <- w404
        n194 = Interpolate 1D Array ("一维数组插值")(1:"S棒组", 2:w413) -> (0:w402:dbl)
        "S棒价值" <- w402
        n195 = Interpolate 1D Array(1:"A棒组", 2:w418) -> (0:w403:dbl)
        "A棒价值" <- w403
        n196 = Multiply(x=w410, y="硼浓度 (ppm)") -> (x*y=w391:dbl)
        "硼总价值 (pcm)" <- w391
        n197 = Build Array("硼浓度 (ppm)", "D棒组", "C棒组", "B棒组", "A棒组", "S棒组") -> (→"棒位与硼浓度":dbl[])
        n198 = Build Array(w406, w405, w404, w403, w402) -> (w417:dbl[])
        n199 = Add Array Elements(numeric array=w417) -> (sum=w392:dbl)
        "棒总价值 (pcm)" <- w392
        n200 = Add(x=w391, y=w392) -> (x+y=w407:dbl)
        n201 = Add(x=w407, y="堆芯后备反应性 (pcm)") -> (x+y=w394:dbl)
        "堆芯反应性(硼+棒) (pcm)" <- w394
        n202 = Multiply(x=1e-05, y=w394) -> (x*y=w415:dbl)
        n203 = Subtract(x=w412, y=w415) -> (x-y=w414:dbl)
        n204 = Divide(x=w412, y=w414) -> (x/y=→"keff":dbl)
        n205 = case shown="True" "反应性控制方式" {
          tunnel: w394 -> [_ w422]
          frame False {
          }
          frame True {
            n206 = local write "堆芯反应性 (pcm)"(w422) -> ()
          }
        }
        "硼浓度 indicator" <- "硼浓度 (ppm)"
      }
      event "停止": Value Change {
        n207 = event-data() -> ()  [unwired: 1 in, 6 out]
        n208 = local read "停止"() -> (w423:bool)
      }
    }
  }
  n209 = Not Equal?(x=w6, y=w11) -> (x != y?=w7:bool)
  n210 = And(x=w9, y=w10) -> (x .and. y?=w5:bool)
  n211 = while {
    tunnel: w162 -> [w512]
    tunnel: w160 -> [w489]
    tunnel: w146 -> [w508]
    tunnel: w145 -> [w507]
    tunnel: [w506] -> w140
    tunnel: [w505] -> w141
    tunnel: w77 -> [w488]
    tunnel: w63 -> [w484]
    tunnel: w62 -> [w440]
    tunnel: w61 -> [w441]
    tunnel: [w461] -> w22
    tunnel: [w446] -> w23
    tunnel: w60 -> [w437]
    tunnel: [w443] -> w59
    tunnel: w44 -> [w459]
    i -> [w511]
    stop <- "停止" stop-if-true
    w433 = u16[] []  # U16 整型
    w435 = 0.0 ("元素")
    w460 = FALSE  # 1-5V/0-10V
    w476 = 0.001 ("y")
    w479 = 1e-13 ("y")
    # "电流仪器值传入网络"
    # "仪器值，传入网络"
    # "源量程一式三份"
    n212 = Divide(x=w488, y=10000.0) -> (x/y=w487:dbl)
    n213 = Multiply(x=w489, y=w511) -> (x*y=w429:dbl)
    "运行时间 (s)" <- w429
    n214 = Multiply(x=w489, y=1000.0) -> (x*y=w491:dbl)
    n215 = case shown="True" w437 {
      tunnel: w441 -> [w527 w535]
      tunnel: [w527 w534] -> w438
      tunnel: w440 -> [w528 w533]
      tunnel: [w528 w533] -> w439
      tunnel: [sgl[] [] ("单精度浮点") w529] -> w426
      frame False {
      }
      frame True {
        w532 = u16 8  # Quantity
        w536 = u16 0  # Address
        n216 = call-poly "MB Slave Operations (poly).vi"("Starting Address"=w536, "Quantity"=w532, "error in"=w535) -> ("Holding Registers"=w531:u16[], "error out"=w534:errorcluster)  [unwired: 1 in, 14 out]
        n217 = Type Cast(type=sgl[] [] ("单精度浮点"), x=w531) -> (*(type *) &x=w529:sgl[])
      }
    }
    "反应性仪输出电压" <- w426
    n218 = Add(x=w484, y=u16 1) -> (x+y=w470:u16)
    n219 = Multiply(x=1e-05, y="堆芯反应性 (pcm)") -> (x*y=w502:dbl)
    n220 = Divide(x=w491, y="时间比例尺") -> (x/y=w493:dbl)
    n221 = dll-call lib="D:/LVprojects/PointReactorSimulator/PointReactorDll.dll" fn="ProcessLoop"(error in=w512, "reactivity"=w502, "nmin"=w487) -> ("nflux"=w495:dbl)  [unwired: 2 in, 4 out]
    n222 = Wait (ms)(milliseconds to wait=w493) -> ()  [unwired: 1 out]
    n223 = Multiply(x=w495, y=1.0) -> (x*y=w428:dbl)
    "中子注量率" <- w428
    "中子注量曲线" <- w428
    "中子注量率 (n/cm2·s)" <- w428
    n224 = local read "棒位与硼浓度"() -> (w469:dbl[])
    n225 = Multiply(x=2e-08 ("y"), y=w428) -> (x*y=→"%FP":dbl)
    n226 = Multiply(x=8.0 ("y"), y=w428) -> (x*y=w458:dbl)
    "源量程 (CPS)" <- w458
    n227 = Multiply(x=8e-14 ("y"), y=w428) -> (x*y=w430:dbl)
    "中间量程 (A)" <- w430
    n228 = Index Array(array=w469) -> (element #1=w463:dbl, element #2=w468:dbl, element #3=w467:dbl, element #4=w466:dbl, element #5=w465:dbl, element #6=w464:dbl)  [unwired: 6 in]
    n229 = Multiply(x=2.3e-14 ("y"), y=w428) -> (x*y=w431:dbl)
    "功率量程 (A)" <- w431
    n230 = Build Array(w458, w458, w458) -> (w457:dbl[])
    n231 = Build Array(w468, w467, w466, w465, w464, w463, w430, w458) -> (w453:dbl[])
    n232 = Build Array(w430, w431, w435, w435) -> (w455:dbl[])
    n233 = Index Array(array=w469, index #1=0 ("索引"), index #2=w470) -> (element #1=w473:dbl, element #2=w472:dbl)
    n234 = for {
      tunnel: w453 -> [w632] mode=indexing
      tunnel: [w631] -> w456 mode=indexing
      tunnel: w460 -> [w633]
      tunnel: w459 -> [w630] mode=indexing
      n235 = case shown="False" w633 {
        tunnel: w632 -> [w636 w675]
        tunnel: [w635 w674] -> w631
        tunnel: w630 -> [w634 w673]
        frame False {
          n236 = case shown="2" w634 {
            tunnel: w636 -> [w639 w646 w652 w655 w662 w669]
            tunnel: [w637 w645 w652 w653 w660 w667] -> w635
            frame 3 {
              # "温度"
              n237 = Subtract(x=w639, y=275.0) -> (x-y=w640:dbl)
              n238 = Multiply(x=w640, y=4.0) -> (x*y=w642:dbl)
              n239 = Divide(x=w642, y=60.0) -> (x/y=w638:dbl)
              n240 = Increment(x=w638) -> (x+1=w637:dbl)
            }
            frame 4 {
              # "硼浓度"
              n241 = Multiply(x=4.0, y=w646) -> (x*y=w648:dbl)
              n242 = Divide(x=w648, y=2000.0) -> (x/y=w650:dbl)
              n243 = Add(x=w650, y=1.0) -> (x+y=w645:dbl)
            }
            frame Default {
            }
            frame 0 {
              # "源量程脉冲"
              n244 = Logarithm Base 10(1:w655) -> (0:w656:dbl)
              n245 = Multiply(x=w656, y=4.0) -> (x*y=w659:dbl)
              n246 = Divide(x=w659, y=7.0) -> (x/y=w654:dbl)
              n247 = Increment(x=w654) -> (x+1=w653:dbl)
            }
            frame 1 {
              # "中间量程电流"
              n248 = Logarithm Base 10(1:w662) -> (0:w663:dbl)
              n249 = Add(x=w663, y=11.0) -> (x+y=w666:dbl)
              n250 = Divide(x=w666, y=2.0) -> (x/y=w661:dbl)
              n251 = Increment(x=w661) -> (x+1=w660:dbl)
            }
            frame 2 {
              # "棒位"
              n252 = Multiply(x=w669, y=4.0) -> (x*y=w671:dbl)
              n253 = Divide(x=w671, y=225.0) -> (x/y=w668:dbl)
              n254 = Increment(x=w668) -> (x+1=w667:dbl)
            }
          }
        }
        frame True {
          n255 = case shown="2" w673 {
            tunnel: w675 -> [w677 w684 w688 w690 w696 w702]
            tunnel: [w676 w683 w688 w689 w695 w701] -> w674
            frame 3 {
              # "温度"
              n256 = Subtract(x=w677, y=275.0) -> (x-y=w678:dbl)
              n257 = Multiply(x=w678, y=10.0) -> (x*y=w680:dbl)
              n258 = Divide(x=w680, y=60.0) -> (x/y=w676:dbl)
            }
            frame 4 {
              # "硼浓度"
              n259 = Multiply(x=10.0, y=w684) -> (x*y=w686:dbl)
              n260 = Divide(x=w686, y=2000.0) -> (x/y=w683:dbl)
            }
            frame Default {
            }
            frame 0 {
              # "源量程脉冲"
              n261 = Logarithm Base 10(1:w690) -> (0:w691:dbl)
              n262 = Multiply(x=w691, y=10.0) -> (x*y=w694:dbl)
              n263 = Divide(x=w694, y=7.0) -> (x/y=w689:dbl)
            }
            frame 1 {
              # "中间量程电流"
              n264 = Logarithm Base 10(1:w696) -> (0:w697:dbl)
              n265 = Add(x=w697, y=11.0) -> (x+y=w700:dbl)
              n266 = Divide(x=w700, y=0.8) -> (x/y=w695:dbl)
            }
            frame 2 {
              # "棒位"
              n267 = Multiply(x=w702, y=10.0) -> (x*y=w704:dbl)
              n268 = Divide(x=w704, y=235.0) -> (x/y=w701:dbl)
            }
          }
        }
      }
    }
    n269 = Build Array (concatenate)(w457, w456, w455) -> (w454:dbl[])
    n270 = Build Array(w430, w431) -> (w482:dbl[])
    n271 = Index Array(array=w482, index="电流输出选择") -> (element=w478:dbl)
    n272 = Greater Or Equal?(x=w478, y=w479) -> (x >= y?=w480:bool)
    n273 = Select(t=w478, s=w480, f=w479) -> (s? t:f=w475:dbl)
    n274 = Less Or Equal?(x=w475, y=w476) -> (x <= y?=w477:bool)
    n275 = Select(t=w475, s=w477, f=w476) -> (s? t:f=w474:dbl)
    n276 = Build Array(w429, w458, "堆芯反应性 (pcm)", w430, "堆芯反应性 (pcm)", w431, "堆芯反应性 (pcm)", w473, w472, nan ("元素")) -> (w504:dbl[])
    n277 = local write "输出电流 (A)"(w474) -> ()
    n278 = To Single Precision Float(number=w454) -> (single precision float=w436:sgl[])
    n279 = Type Cast(type=w433, x=w436) -> (*(type *) &x=w434:u16[])
    n280 = case shown="True" "endian Switch" {
      tunnel: w434 -> [w514 w517]
      tunnel: [w514 w515] -> w432
      frame False {
      }
      frame True {
        n281 = for {
          N: 15 -> [_]
          shift-right: [w518] -> w515
          shift-left: w517 -> [w523]
          i -> [w525]
          n282 = Multiply(x=2, y=w525) -> (x*y=w522:i32)
          n283 = Increment(x=w522) -> (x+1=w521:i32)
          n284 = Index Array(array=w523, index #1=w522, index #2=w521) -> (element #1=w520:u16, element #2=w519:u16)
          n285 = Replace Array Subset(array=w523, new element #1=w519, index #1=w522, new element #2=w520, index #2=w521) -> (w518:u16[])
        }
      }
    }
    n286 = case shown="True" w437 {
      tunnel: w438 -> [w707 w713]
      tunnel: [w707 w712] -> w446
      tunnel: w439 -> [w708 w711]
      tunnel: [w708 w711] -> w461
      tunnel: [FALSE TRUE] -> w443
      tunnel: w432 -> [_ w709]
      frame False {
      }
      frame True {
        n287 = call-poly "MB Slave Operations (poly).vi"("Starting Address"=u16 0 ("Address"), "Input Registers"=w709, "error in"=w713) -> ("error out"=w712:errorcluster)  [unwired: 1 in, 15 out]
      }
    }
    n288 = Build Array("VO 1", "VO 2", "VO 3", "VO 4") -> (w448:u16[])
    n289 = for {
      N: 4 -> [_]
      tunnel: w453 -> [w539]
      tunnel: [w540] -> w425 mode=indexing
      tunnel: "电压输出选择" -> [w541]
      tunnel: w448 -> [w537] mode=indexing
      n290 = Index Array(array=w539, index=w537) -> (element=w538:dbl)
      n291 = case shown="True" w541 {
        tunnel: w538 -> [w544 w599]
        tunnel: [w543 w598] -> w540
        tunnel: w537 -> [w542 w597]
        frame False {
          n292 = case shown="3" w542 {
            tunnel: w544 -> [w546 w552 w558 w561 w568 w575 w580 w586 w592]
            tunnel: [w545 w551 w558 w559 w566 w573 w579 w585 w591] -> w543
            frame 4 {
              # "棒位"
              n293 = Multiply(x=w546, y=4.0) -> (x*y=w549:dbl)
              n294 = Divide(x=w549, y=225.0) -> (x/y=w547:dbl)
              n295 = Increment(x=w547) -> (x+1=w545:dbl)
            }
            frame 5 {
              # "硼浓度"
              n296 = Multiply(x=4.0, y=w552) -> (x*y=w554:dbl)
              n297 = Divide(x=w554, y=2000.0) -> (x/y=w556:dbl)
              n298 = Add(x=w556, y=1.0) -> (x+y=w551:dbl)
            }
            frame Default {
            }
            frame 7 {
              # "源量程脉冲"
              n299 = Logarithm Base 10(1:w561) -> (0:w562:dbl)
              n300 = Multiply(x=w562, y=4.0) -> (x*y=w565:dbl)
              n301 = Divide(x=w565, y=7.0) -> (x/y=w560:dbl)
              n302 = Increment(x=w560) -> (x+1=w559:dbl)
            }
            frame 6 {
              # "中间量程电流"
              n303 = Logarithm Base 10(1:w568) -> (0:w569:dbl)
              n304 = Add(x=w569, y=11.0) -> (x+y=w572:dbl)
              n305 = Divide(x=w572, y=2.0) -> (x/y=w567:dbl)
              n306 = Increment(x=w567) -> (x+1=w566:dbl)
            }
            frame 0 {
              # "棒位"
              n307 = Multiply(x=w575, y=4.0) -> (x*y=w577:dbl)
              n308 = Divide(x=w577, y=225.0) -> (x/y=w574:dbl)
              n309 = Increment(x=w574) -> (x+1=w573:dbl)
            }
            frame 1 {
              # "棒位"
              n310 = Multiply(x=w580, y=4.0) -> (x*y=w583:dbl)
              n311 = Divide(x=w583, y=225.0) -> (x/y=w581:dbl)
              n312 = Increment(x=w581) -> (x+1=w579:dbl)
            }
            frame 2 {
              # "棒位"
              n313 = Multiply(x=w586, y=4.0) -> (x*y=w589:dbl)
              n314 = Divide(x=w589, y=225.0) -> (x/y=w587:dbl)
              n315 = Increment(x=w587) -> (x+1=w585:dbl)
            }
            frame 3 {
              # "棒位"
              n316 = Multiply(x=w592, y=4.0) -> (x*y=w595:dbl)
              n317 = Divide(x=w595, y=225.0) -> (x/y=w593:dbl)
              n318 = Increment(x=w593) -> (x+1=w591:dbl)
            }
          }
        }
        frame True {
          n319 = case shown="3" w597 {
            tunnel: w599 -> [w601 w608 w612 w614 w620 w626]
            tunnel: [w600 w607 w612 w613 w619 w625] -> w598
            frame 3 {
              # "温度"
              n320 = Subtract(x=w601, y=275.0) -> (x-y=w602:dbl)
              n321 = Multiply(x=w602, y=10.0) -> (x*y=w604:dbl)
              n322 = Divide(x=w604, y=60.0) -> (x/y=w600:dbl)
            }
            frame 4 {
              # "硼浓度"
              n323 = Multiply(x=10.0, y=w608) -> (x*y=w610:dbl)
              n324 = Divide(x=w610, y=2000.0) -> (x/y=w607:dbl)
            }
            frame Default {
            }
            frame 0 {
              # "源量程脉冲"
              n325 = Logarithm Base 10(1:w614) -> (0:w615:dbl)
              n326 = Multiply(x=w615, y=10.0) -> (x*y=w618:dbl)
              n327 = Divide(x=w618, y=7.0) -> (x/y=w613:dbl)
            }
            frame 1 {
              # "中间量程电流"
              n328 = Logarithm Base 10(1:w620) -> (0:w621:dbl)
              n329 = Add(x=w621, y=11.0) -> (x+y=w624:dbl)
              n330 = Divide(x=w624, y=0.8) -> (x/y=w619:dbl)
            }
            frame 2 {
              # "棒位"
              n331 = Multiply(x=w626, y=10.0) -> (x*y=w628:dbl)
              n332 = Divide(x=w628, y=225.0) -> (x/y=w625:dbl)
            }
          }
        }
      }
    }
    "输出电压" <- w425
    n333 = Array To Spreadsheet String(array=w504, 3:"%g" ("format string")) -> (spreadsheet string=w503:string)  [unwired: 1 in]
    n334 = Unbundle By Name(w446) -> ("status"=w445:bool)
    n335 = Not(x=w445) -> (.not. x?=w444:bool)
    n336 = And(x=w443, y=w444) -> (x .and. y?=w442:bool)
    n337 = local write "TCP服务器开"(w442) -> ()
    n338 = Write to Binary File(file (use dialog)=w508, data=w503, error in=w507, 5:FALSE ("预置数组或字符串大小？(T)")) -> (refnum out=w506:refnum<file>, error out=w505:errorcluster)  [unwired: 2 in, 1 out]
  }
  n339 = case shown="True" w39 {
    tunnel: u32 1500 ("timeout (10sec)") -> [_ w727]
    tunnel: w42 -> [_ w721]
    tunnel: w33 -> [_ w720]
    tunnel: w40 -> [_ w719]
    tunnel: [errorcluster {"status"=FALSE, "code"=0, "source"=""} ("error out") w718] -> w30
    tunnel: [FALSE ("status") FALSE ("status")] -> w27
    frame False {
    }
    frame True {
      n340 = call-poly "VISA Configure Serial Port"("VISA resource name"=w719, "timeout (10sec)"=w727, "Enable Termination\nChar (T)"=FALSE ("Termination(T)"), "baud rate (9600)"=w720) -> ("VISA resource name out"=w726:refnum<visa-resource-name>, "error out"=w725:errorcluster)  [unwired: 5 in, 5 out]
      n341 = while {
        tunnel: w726 -> [w748]
        tunnel: w725 -> [w747]
        tunnel: [w742] -> w723
        tunnel: [w736] -> w722
        tunnel: w721 -> [w741]
        stop <- w735 stop-if-true
        n342 = property class="Instr"(reference=w748, error in=w747) -> (reference out=w745:refnum<visa-resource-name>, error out=w746:errorcluster, "Serial Settings:Number of Bytes at Serial Port"=w731:u32)
        n343 = Greater Or Equal?(x=w731, y=u32 6) -> (x >= y?=w729:bool)
        n344 = case shown="False" w729 {
          tunnel: w746 -> [w750 w762]
          tunnel: w745 -> [w751 w761]
          tunnel: [w750 w760] -> w744
          tunnel: [w751 w759] -> w743
          tunnel: w741 -> [_ w757]
          tunnel: w731 -> [_ w758]
          tunnel: [-1 w753] -> w740
          frame False {
          }
          frame True {
            n345 = VISA Read(VISA resource name=w761, byte count=w758, error in (no error)=w762) -> (VISA resource name out=w759:refnum<visa-resource-name>, read buffer=w756:string, error out=w760:errorcluster)  [unwired: 1 out]
            n346 = for {
              tunnel: w757 -> [w766] mode=indexing
              tunnel: w756 -> [w767]
              tunnel: [w764] -> w754
              tunnel: [w763] -> w755
              i -> [w764]
              stop <- w763 stop-if-true
              n347 = Search/Split String(string=w767, search string/char (-)=w766) -> (offset of match=w765:i32)  [unwired: 1 in, 2 out]
              n348 = Greater Or Equal To 0?(x=w765) -> (x >= 0?=w763:bool)
            }
            n349 = Select(t=w754, s=w755, f=-1) -> (s? t:f=w753:i32)
          }
        }
        n350 = local read "功率量程 (A)"() -> (w737:dbl)
        n351 = case shown="2" w740 {
          tunnel: [w769 w777 w779 w791] -> w736
          tunnel: w743 -> [w768 w776 w782 w790]
          tunnel: w744 -> [w769 w775 w780 w789]
          tunnel: [w768 w774 w781 w792] -> w742
          tunnel: w737 -> [_ w771 _ w788]
          tunnel: 0 ("Integer32") -> [_ w770 _ _]
          tunnel: "KEITHLEY INSTRUMENTS INC.,MODEL 6485,4084828,C01   Jun 23 2010 12:22:00//H\r" ("y") -> [_ _ w778 _]
          frame -1, Default {
          }
          frame 0 {
            n352 = To Single Precision Float(number=w771) -> (single precision float=w773:sgl)
            n353 = call "Sti_Switch.vi"("Integer32"=w770, "自定义浮点32"=w773) -> ("20B_StrOut"=w772:string)  [unwired: 9 in]
            n354 = VISA Write(VISA resource name=w776, write buffer=w772, error in (no error)=w775) -> (VISA resource name out=w774:refnum<visa-resource-name>, error out=w777:errorcluster)  [unwired: 1 out]
          }
          frame 1 {
            n355 = VISA Write(VISA resource name=w782, write buffer=w778, error in (no error)=w780) -> (VISA resource name out=w781:refnum<visa-resource-name>, error out=w779:errorcluster)  [unwired: 1 out]
          }
          frame 2 {
            n356 = Number To Exponential String(number=w788, precision (6)=i16 6 ("精度(6)"), 3:i16 13 ("宽度(-)")) -> (E-format string=w785:string)  [unwired: 1 in]
            n357 = Concatenate Strings(w785, "\r" ("字符串")) -> (w784:string)
            n358 = VISA Write(VISA resource name=w790, write buffer=w784, error in (no error)=w789) -> (VISA resource name out=w792:refnum<visa-resource-name>, error out=w791:errorcluster)  [unwired: 1 out]
          }
        }
        n359 = local read "停止"() -> (w734:bool)
        n360 = Unbundle By Name(w736) -> ("status"=w733:bool)
        n361 = Not(x=w733) -> (.not. x?=→"COM1":bool)
        n362 = Or(x=w733, y=w734) -> (x .or. y?=w735:bool)
      }
      n363 = VISA Close(VISA resource name=w723, error in (no error)=w722) -> (error out=w724:errorcluster)
      n364 = call <vilib>:"Simple Error Handler.vi"("error in (no error)"=w724) -> ("error out"=w718:errorcluster)  [unwired: 1 in, 7 out]
    }
  }
  n365 = case shown="True" w34 {
    tunnel: w42 -> [_ w799]
    tunnel: w38 -> [_ w798]
    tunnel: w33 -> [_ w797]
    tunnel: [errorcluster {"status"=FALSE, "code"=0, "source"=""} ("error out") w796] -> w29
    tunnel: [FALSE ("status") FALSE ("status")] -> w26
    frame False {
    }
    frame True {
      n366 = call-poly "VISA Configure Serial Port"("VISA resource name"=w798, "timeout (10sec)"=u32 1500, "Enable Termination\nChar (T)"=FALSE ("Termination(T)"), "baud rate (9600)"=w797) -> ("VISA resource name out"=w802:refnum<visa-resource-name>, "error out"=w803:errorcluster)  [unwired: 5 in, 5 out]
      n367 = while {
        tunnel: w802 -> [w826]
        tunnel: w803 -> [w825]
        tunnel: [w820] -> w805
        tunnel: [w814] -> w806
        tunnel: w799 -> [w819]
        stop <- w813 stop-if-true
        n368 = property class="Instr"(reference=w826, error in=w825) -> (reference out=w823:refnum<visa-resource-name>, error out=w824:errorcluster, "Serial Settings:Number of Bytes at Serial Port"=w808:u32)
        n369 = Greater Or Equal?(x=w808, y=u32 6) -> (x >= y?=w807:bool)
        n370 = case shown="True" w807 {
          tunnel: w824 -> [w828 w840]
          tunnel: w823 -> [w829 w839]
          tunnel: [w828 w838] -> w822
          tunnel: [w829 w837] -> w821
          tunnel: w819 -> [_ w835]
          tunnel: w808 -> [_ w836]
          tunnel: [-1 w831] -> w818
          frame False {
          }
          frame True {
            n371 = VISA Read(VISA resource name=w839, byte count=w836, error in (no error)=w840) -> (VISA resource name out=w837:refnum<visa-resource-name>, read buffer=w834:string, error out=w838:errorcluster)  [unwired: 1 out]
            n372 = for {
              tunnel: w835 -> [w844] mode=indexing
              tunnel: w834 -> [w845]
              tunnel: [w842] -> w832
              tunnel: [w841] -> w833
              i -> [w842]
              stop <- w841 stop-if-true
              n373 = Search/Split String(string=w845, search string/char (-)=w844) -> (offset of match=w843:i32)  [unwired: 1 in, 2 out]
              n374 = Greater Or Equal To 0?(x=w843) -> (x >= 0?=w841:bool)
            }
            n375 = Select(t=w832, s=w833, f=-1) -> (s? t:f=w831:i32)
          }
        }
        n376 = local read "中间量程 (A)"() -> (w815:dbl)
        n377 = case shown="2" w818 {
          tunnel: [w847 w855 w857 w869] -> w814
          tunnel: w821 -> [w846 w854 w860 w868]
          tunnel: w822 -> [w847 w853 w858 w867]
          tunnel: [w846 w852 w859 w870] -> w820
          tunnel: w815 -> [_ w849 _ w866]
          tunnel: 0 ("Integer32") -> [_ w848 _ _]
          tunnel: "KEITHLEY INSTRUMENTS INC.,MODEL 6485,4084828,C01   Jun 23 2010 12:22:00//H\r" ("y") -> [_ _ w856 _]
          frame -1, Default {
          }
          frame 0 {
            n378 = To Single Precision Float(number=w849) -> (single precision float=w851:sgl)
            n379 = call "Sti_Switch.vi"("Integer32"=w848, "自定义浮点32"=w851) -> ("20B_StrOut"=w850:string)  [unwired: 9 in]
            n380 = VISA Write(VISA resource name=w854, write buffer=w850, error in (no error)=w853) -> (VISA resource name out=w852:refnum<visa-resource-name>, error out=w855:errorcluster)  [unwired: 1 out]
          }
          frame 1 {
            n381 = VISA Write(VISA resource name=w860, write buffer=w856, error in (no error)=w858) -> (VISA resource name out=w859:refnum<visa-resource-name>, error out=w857:errorcluster)  [unwired: 1 out]
          }
          frame 2 {
            n382 = Number To Exponential String(number=w866, precision (6)=i16 6 ("精度(6)"), 3:i16 13 ("宽度(-)")) -> (E-format string=w863:string)  [unwired: 1 in]
            n383 = Concatenate Strings(w863, "\r" ("字符串")) -> (w862:string)
            n384 = VISA Write(VISA resource name=w868, write buffer=w862, error in (no error)=w867) -> (VISA resource name out=w870:refnum<visa-resource-name>, error out=w869:errorcluster)  [unwired: 1 out]
          }
        }
        n385 = local read "停止"() -> (w812:bool)
        n386 = Unbundle By Name(w814) -> ("status"=w810:bool)
        n387 = Not(x=w810) -> (.not. x?=→"COM2":bool)
        n388 = Or(x=w810, y=w812) -> (x .or. y?=w813:bool)
      }
      n389 = VISA Close(VISA resource name=w805, error in (no error)=w806) -> (error out=w804:errorcluster)
      n390 = call <vilib>:"Simple Error Handler.vi"("error in (no error)"=w804) -> ("error out"=w796:errorcluster)  [unwired: 1 in, 7 out]
    }
  }
  n391 = case shown="True" w7 {
    tunnel: w6 -> [_ w897]
    tunnel: [errorcluster {"status"=FALSE, "code"=0, "source"=""} ("error out") w875] -> w32
    tunnel: [FALSE ("停止") TRUE ("停止")] -> w25
    frame False {
      n392 = property on="电流输出选择" class="Ring (strict)"("DisabledEnum"=T1."Disabled and Grayed Out" ("禁用")) -> ()  [unwired: 2 in, 2 out]
    }
    frame True {
      w889 = T8 {"Auto Range?"=TRUE, "Man / Selected\nRange"=enum."2nA"}  # Current Range In
      w896 = FALSE  # Check For SCPI Errors? (T)
      w893 = FALSE ("Read Back Set Values? (T)")
      n393 = call "Initialize.vi"("VISA resource name"=w897, "Error Queue Option"=enum16{"Clear Error Queue", "Error Query"}."Clear Error Queue", "Instrument Type"=KE622x_--_Instrument_Type."KE6220") -> ("VISA resource name out"=w887:refnum<visa-resource-name>, "error out"=w886:errorcluster)  [unwired: 11 in]
      n394 = property on="电流输出选择" class="Ring (strict)"("DisabledEnum"=T1."Enabled" ("禁用")) -> ()  [unwired: 2 in, 2 out]
      n395 = Boolean To (0,1)(Boolean=FALSE ("布尔")) -> (0, 1=w879:i16)
      n396 = call "KE622x -- Set Analog Filter State.vi"("Resource In"=w887, "Check For SCPI Errors? (T)"=w896, "Analog Filter State"=w879, "error in (no error)"=w886) -> ("Resource Out (dupl)"=w883:refnum<visa-resource-name>, "error out"=w884:errorcluster)  [unwired: 10 in]
      n397 = call "KE622x -- Set Current Range.vi"("Resource In"=w883, "Check For SCPI Errors? (T)"=w896, "Current Range In"=w889, "error in (no error)"=w884, "Read Back Set Values? (T)"=w893) -> ("Resource Out (dupl)"=w881:refnum<visa-resource-name>, "error out"=w880:errorcluster)  [unwired: 8 in, 1 out]
      n398 = call "KE622x -- Set Voltage Limit.vi"("Resource In"=w881, "Check For SCPI Errors? (T)"=w896, "Voltage Limit (V)"=T6 10.0, "error in (no error)"=w880) -> ("Resource Out (dupl)"=w895:refnum<visa-resource-name>, "error out"=w894:errorcluster)  [unwired: 10 in]
      n399 = while {
        tunnel: w896 -> [w913]
        tunnel: w895 -> [w912]
        tunnel: w894 -> [w911]
        tunnel: w893 -> [w910]
        tunnel: [w909] -> w892
        tunnel: [w908] -> w891
        tunnel: [w903] -> w890
        stop <- w900 stop-if-true
        n400 = call "KE622x -- Set Current Level.vi"("Resource In"=w912, "Check For SCPI Errors? (T)"=w913, "Current Level (A) In"="输出电流 (A)", "error in (no error)"=w911, "Read Back Set Value? (T)"=w910) -> ("Resource Out (dupl)"=w907:refnum<visa-resource-name>, "error out"=w906:errorcluster)  [unwired: 8 in, 1 out]
        n401 = Boolean To (0,1)(Boolean=TRUE ("布尔")) -> (0, 1=w905:i16)
        n402 = case shown="0, Default" w905 {
          selector: w905 -> [w917 _]
          tunnel: w907 -> [w919 w925]
          tunnel: w906 -> [w918 w924]
          tunnel: [w916 w922] -> w903
          tunnel: w913 -> [w914 w920]
          tunnel: [w915 w921] -> w908
          tunnel: [w914 w920] -> w909
          frame 0, Default {
            n403 = call "KE622x -- Set Output State.vi"("Resource In"=w919, "Check For SCPI Errors? (T)"=w914, "Output State"=w917, "error in (no error)"=w918) -> ("Resource Out (dupl)"=w915:refnum<visa-resource-name>, "error out"=w916:errorcluster)  [unwired: 10 in]
          }
          frame 1 {
            n404 = call "KE622x -- Turn Output On And Check For Errors.vi"("Resource In"=w925, "Check For SCPI Errors? (T)"=w920, "Turn Off Output If Compliance?"=TRUE ("Turn Off Output\nIf Voltage Limit?"), "error in (no error)"=w924) -> ("Resource Out (dupl)"=w921:refnum<visa-resource-name>, "error out"=w922:errorcluster)  [unwired: 8 in, 2 out]
          }
        }
        n405 = Unbundle By Name(w903) -> ("status"=w899:bool)
        n406 = local read "停止"() -> (w901:bool)
        n407 = Not(x=w899) -> (.not. x?=→"KE6220_1":bool)
        n408 = Or(x=w901, y=w899) -> (x .or. y?=w900:bool)
      }
      n409 = call "Close.vi"("VISA resource name"=w891, "Query For SCPI Errors? (T)"=w892, "error in (no error)"=w890) -> ("error out"=w877:errorcluster)  [unwired: 12 in]
      n410 = call <vilib>:"Simple Error Handler.vi"("error in (no error)"=w877) -> ("error out"=w875:errorcluster)  [unwired: 4 in, 4 out]
    }
  }
  n411 = case shown="True" w5 {
    tunnel: w4 -> [_ w950]
    tunnel: [errorcluster {"status"=FALSE, "code"=0, "source"=""} ("error out") w929] -> w12
    tunnel: [FALSE ("停止") TRUE ("停止")] -> w13
    frame False {
    }
    frame True {
      w942 = T8 {"Auto Range?"=TRUE, "Man / Selected\nRange"=enum."2nA"}  # Current Range In
      w949 = FALSE  # Check For SCPI Errors? (T)
      w946 = FALSE ("Read Back Set Values? (T)")
      n412 = call "Initialize.vi"("VISA resource name"=w950, "Error Queue Option"=enum16{"Clear Error Queue", "Error Query"}."Clear Error Queue", "Instrument Type"=KE622x_--_Instrument_Type."KE6220") -> ("VISA resource name out"=w940:refnum<visa-resource-name>, "error out"=w939:errorcluster)  [unwired: 11 in]
      n413 = Boolean To (0,1)(Boolean=FALSE ("布尔")) -> (0, 1=w932:i16)
      n414 = call "KE622x -- Set Analog Filter State.vi"("Resource In"=w940, "Check For SCPI Errors? (T)"=w949, "Analog Filter State"=w932, "error in (no error)"=w939) -> ("Resource Out (dupl)"=w936:refnum<visa-resource-name>, "error out"=w937:errorcluster)  [unwired: 10 in]
      n415 = call "KE622x -- Set Current Range.vi"("Resource In"=w936, "Check For SCPI Errors? (T)"=w949, "Current Range In"=w942, "error in (no error)"=w937, "Read Back Set Values? (T)"=w946) -> ("Resource Out (dupl)"=w934:refnum<visa-resource-name>, "error out"=w933:errorcluster)  [unwired: 8 in, 1 out]
      n416 = call "KE622x -- Set Voltage Limit.vi"("Resource In"=w934, "Check For SCPI Errors? (T)"=w949, "Voltage Limit (V)"=T6 10.0, "error in (no error)"=w933) -> ("Resource Out (dupl)"=w948:refnum<visa-resource-name>, "error out"=w947:errorcluster)  [unwired: 10 in]
      n417 = while {
        tunnel: w949 -> [w966]
        tunnel: w948 -> [w965]
        tunnel: w947 -> [w964]
        tunnel: w946 -> [w963]
        tunnel: [w962] -> w945
        tunnel: [w961] -> w944
        tunnel: [w956] -> w943
        stop <- w955 stop-if-true
        n418 = local read "输出电流 (A)"() -> (w951:dbl)
        n419 = call "KE622x -- Set Current Level.vi"("Resource In"=w965, "Check For SCPI Errors? (T)"=w966, "Current Level (A) In"=w951, "error in (no error)"=w964, "Read Back Set Value? (T)"=w963) -> ("Resource Out (dupl)"=w960:refnum<visa-resource-name>, "error out"=w959:errorcluster)  [unwired: 8 in, 1 out]
        n420 = Boolean To (0,1)(Boolean=TRUE ("布尔")) -> (0, 1=w958:i16)
        n421 = case shown="0, Default" w958 {
          selector: w958 -> [w970 _]
          tunnel: w960 -> [w972 w978]
          tunnel: w959 -> [w971 w977]
          tunnel: [w969 w975] -> w956
          tunnel: w966 -> [w967 w973]
          tunnel: [w968 w974] -> w961
          tunnel: [w967 w973] -> w962
          frame 0, Default {
            n422 = call "KE622x -- Set Output State.vi"("Resource In"=w972, "Check For SCPI Errors? (T)"=w967, "Output State"=w970, "error in (no error)"=w971) -> ("Resource Out (dupl)"=w968:refnum<visa-resource-name>, "error out"=w969:errorcluster)  [unwired: 10 in]
          }
          frame 1 {
            n423 = call "KE622x -- Turn Output On And Check For Errors.vi"("Resource In"=w978, "Check For SCPI Errors? (T)"=w973, "Turn Off Output If Compliance?"=TRUE ("Turn Off Output\nIf Voltage Limit?"), "error in (no error)"=w977) -> ("Resource Out (dupl)"=w974:refnum<visa-resource-name>, "error out"=w975:errorcluster)  [unwired: 8 in, 2 out]
          }
        }
        n424 = Unbundle By Name(w956) -> ("status"=w954:bool)
        n425 = local read "停止"() -> (w953:bool)
        n426 = Not(x=w954) -> (.not. x?=→"KE6220_2":bool)
        n427 = Or(x=w953, y=w954) -> (x .or. y?=w955:bool)
      }
      n428 = call "Close.vi"("VISA resource name"=w944, "Query For SCPI Errors? (T)"=w945, "error in (no error)"=w943) -> ("error out"=w930:errorcluster)  [unwired: 12 in]
      n429 = call <vilib>:"Simple Error Handler.vi"("error in (no error)"=w930) -> ("error out"=w929:errorcluster)  [unwired: 4 in, 4 out]
    }
  }
  n430 = while {
    stop <- w979 stop-if-true
    n431 = event shown="[0] \"归零\": Value Change" {
      selector: _ -> [_ _ _]
      dyn-events: _ -> [_ _ _]
      timeout: _ -> [_ _ _]
      tunnel: [_ _ w990] -> w979
      event "归零": Value Change {
        n432 = event-data() -> ()  [unwired: 1 in, 6 out]
        n433 = disable-structure shown="Disabled" {
          frame Disabled {
            w985 = 0.0 ("堆芯反应性 (pcm)")
            n434 = local write "堆芯反应性(硼+棒) (pcm)"(w985) -> ()
            n435 = local write "堆芯反应性 (pcm)"(w985) -> ()
          }
          frame Enabled {
          }
        }
        n436 = local read "硼总价值 (pcm)"() -> (w983:dbl)
        n437 = local read "棒总价值 (pcm)"() -> (w984:dbl)
        n438 = Add(x=w983, y=w984) -> (x+y=w982:dbl)
        n439 = Subtract(x=0.0, y=w982) -> (x-y=w980:dbl)
        n440 = property on="堆芯后备反应性 (pcm)" class="DigNum (strict)"("Val(Sgnl)"=w980) -> ()  [unwired: 2 in, 2 out]
      }
      event "反应性控制方式": Value Change {
        n441 = event-data() -> ("NewVal"=w986:bool)  [unwired: 1 in, 5 out]
        n442 = case shown="True" w986 {
          frame False {
            n443 = property on="堆芯反应性 (pcm)" class="DigNum (strict)"("DisabledEnum"=T1."Enabled" ("Disabled")) -> ()  [unwired: 2 in, 2 out]
          }
          frame True {
            n444 = local read "堆芯反应性(硼+棒) (pcm)"() -> (w989:dbl)
            n445 = local write "堆芯反应性 (pcm)"(w989) -> ()
            n446 = property on="堆芯反应性 (pcm)" class="DigNum (strict)"("DisabledEnum"=T1."Disabled" ("Disabled")) -> ()  [unwired: 2 in, 2 out]
          }
        }
      }
      event "停止": Value Change {
        n447 = event-data() -> ()  [unwired: 1 in, 6 out]
        n448 = local read "停止"() -> (w990:bool)
      }
    }
  }
  n449 = local write "CARD"(w24) -> ()
  n450 = flat-sequence {
    tunnel: [w993] -> w21
    tunnel: w23 -> [w993]
    tunnel: [w991] -> w20
    tunnel: w22 -> [w991]
    frame #0 {
      n451 = global write "MB Globals.vi" "Ethernet Demon Running"(FALSE ("Slave Demon Running")) -> ()
    }
  }
  n452 = local write "COM2"(w26) -> ()
  n453 = local write "COM1"(w27) -> ()
  n454 = local write "KE6220_1"(w25) -> ()
  n455 = local write "KE6220_2"(w13) -> ()
  n456 = Array To Spreadsheet String(array=string[] ["开始时间：", "00：00", "结束时间：", "00：00"] ("添加的数组"), 3:"%s" ("format string")) -> (spreadsheet string=w138:string)  [unwired: 1 in]
  n457 = Write to Binary File(file (use dialog)=w140, data=w138, error in=w141, 5:FALSE ("预置数组或字符串大小？(T)")) -> (refnum out=w144:refnum<file>, error out=w143:errorcluster)  [unwired: 2 in, 1 out]
  n458 = case shown="True" w59 {
    tunnel: w20 -> [_ w995]
    tunnel: w21 -> [_ w994]
    frame False {
    }
    frame True {
      n459 = Close Reference "关闭引用"(reference=w995, error in (no error)=w994) -> (error out=w996:errorcluster)
      n460 = call <vilib>:"Simple Error Handler.vi"("error in (no error)"=w996) -> ()  [unwired: 1 in, 8 out]
    }
  }
  n461 = flat-sequence {
    tunnel: w144 -> [w999]
    tunnel: w143 -> [w998]
    tunnel: w32 -> [_]
    tunnel: w31 -> [_]
    tunnel: w30 -> [_]
    tunnel: w29 -> [_]
    tunnel: w12 -> [_]
    tunnel: [w997] -> w2
    tunnel: w2 -> [w1000]
    frame #0 {
      n462 = Close File(refnum=w999, error in=w998) -> ()  [unwired: 2 out]
      n463 = property class="App"() -> ("App.Kind"=w997:T10)  [unwired: 2 in, 2 out]
    }
    frame #1 {
      n464 = case shown="\"Run Time System\"" w1000 {
        frame "Development System", Default {
        }
        frame "Run Time System" {
          n465 = invoke class="VI" method="FP.Close"() -> (reference out=w1001:refnum<vi>, error out=w1002:errorcluster)  [unwired: 3 in, 1 out]
          n466 = Close Reference(reference=w1001, error in (no error)=w1002) -> ()  [unwired: 1 out]
        }
      }
    }
  }
